vi "ESP30xCore.vi"(5 "NumOfAxis":i32=3, 6 "MotorDisabled":refnum<vi>, 7 "Simulation":bool, 8 "error in":errorcluster, 9 "Serial Configuration":T1={"Baud Rate"=19200, "Parity"=0, "Data Bits"=8, "Stop Bits"=10, "Flow Control"=2} {"Flow Control" items=["None", "XON/XOFF", "RTS/CTS", "XON/XOFF & RTS/CTS", "DTR/DSR", "XON/XOFF & DTR/DSR"]; "Stop Bits" items=["1.0"=10, "1.5"=15, "2.0"=20]; "Data Bits" items=["7"=7, "8"=8]; "Parity" items=["None", "Odd", "Even", "Mark", "Space"]; "Baud Rate" items=["300"=300, "600"=600, "1200"=1200, "2400"=2400, "4800"=4800, "9600"=9600, "19200"=19200]}, 10 "CommPort":refnum<visa-resource-name>="COM3", 11 "ControlQueue in":refnum<queue>) -> (0 "error out":errorcluster, 3 "queue out":refnum<queue>)   [LabVIEW 2013, in "ESP300.lvlib"]
uses:
  <instrlib>/ESP300/ESP300.lvlib
  <instrlib>/ESP300/Public/Data/ESP300_State.ctl
  <instrlib>/ESP300/Public/Data/ESP30x_Data.ctl
  <vilib>/Utility/error.llb/DialogType.ctl
  <instrlib>/Micos_uic/Public/Data/Micos_State.ctl
  <instrlib>/Micos_uic/Public/Data/Micos_Data.ctl
  <instrlib>/ESP300/Public/Position_ESP300.vi
  <instrlib>/Micos_uic/Micos_uic.lvlib
panel:
  in  "+Z_fine":bool
  in  "-Z_fine":bool
  in  "++Z":bool
  in  "--Z":bool
  in  "+Z":bool
  in  "-Z":bool
  out "WaitStopBlink":i32
  in  "StepWidth":dbl(ring)=0.2 items=["0.2 um"=0.0002, "0.001 mm"=0.001, "0.002 mm"=0.002, "0.005 mm "=0.005, "0.01 mm"=0.01, "0.02 mm"=0.02, "0.05 mm"=0.05, "0.1 mm"=0.1, "0.2 mm"=0.2, "1 mm"=1.0]
  in  "MotorDisabled":bool caption="Go"
  in  "Home":bool caption="Go"
  in  "Z-":bool
  in  "Z+":bool
  in  "X+":bool
  in  "X-":bool
  in  "Y-":bool
  in  "Y+":bool
  in  "ClearErr":bool caption="Go"
  in  "STOP":bool caption="Go"
  in  "Quit":bool caption="Go"
  out "Instrument Driver Revision":string
  out "Instrument Firmware Revision":string
  in  "SetPosition":dbl[](array[numeric])=[10.93352, 0.3355, 20.38401000000006] caption="Position" format="%.4f"
  in  "SetVelocity":dbl[](array[numeric])=[0.2, 0.2, 0.2] caption="Velocity"
  in  "SetAcceleration":dbl[](array[numeric])=[0.8, 0.8, 0.8] caption="Acceleration"
  in  "Go":bool
  out "Moving":bool
  out "Acceleration":dbl[](array[numeric])
  out "Velocity":dbl[](array[numeric])
  out "Position":dbl[](array[numeric])
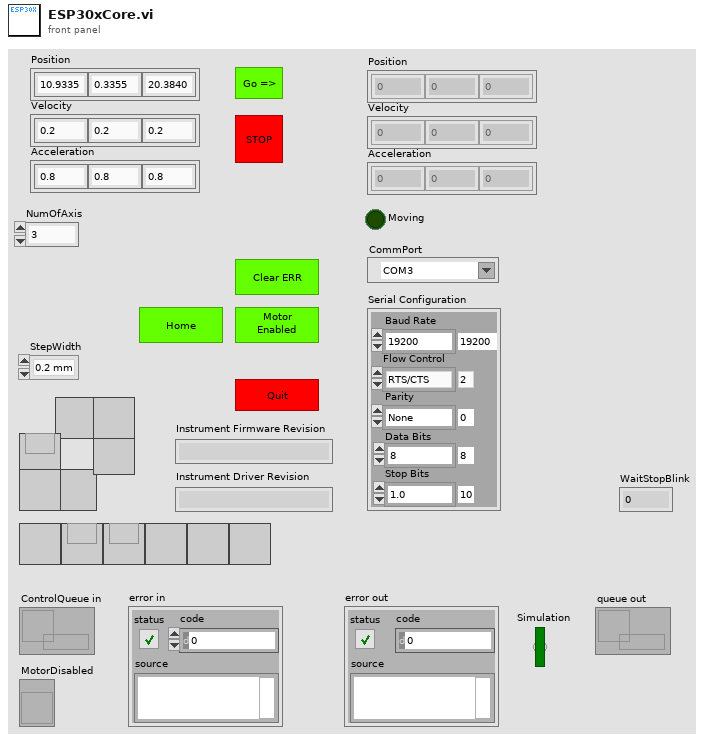
[diagram p1: front panel]
types:
  T1 = cluster{"Baud Rate":u32, "Parity":u16, "Data Bits":u16, "Stop Bits":u16, "Flow Control":u16}
  T2 = cluster{"CommPort":refnum<vi>, "Serial Configuration":refnum<vi>, "SetPosition":refnum<vi>, "SetAcceleration":refnum<vi>, "SetVelocity":refnum<vi>, "StepWidth":refnum<vi>}
  T3 = typedef "ESP300.lvlib/ESP300_State.ctl" = cluster{"State":enum16{"Initialize", "SetDefaultConfig", "Close", "Quit", "Identify", "MoveAbs", "MoveAbs_all", "MoveRel", "MoveRel_all", "STOP", "Origin/Home", "WaitStop", "QueryStatus", "UpdateXPos", "UpdateAll", "SetVelocity", "SetAcceleration", "ClearErr", "LogMessage", "MotorEnable(1)", "EnableAxis", "JoyStick", "GetVelocity", "GetAcceleration", "SendCmd", "SetSoftLimits", "Beep", "_SettingReturn", "SoftReset"}, "Params.":variant}
  T4 = typedef "ESP300.lvlib/ESP30x_Data.ctl" = cluster{"Position":dbl[], "Velocity":dbl[], "Acceleration":dbl[], "Moving":bool, "Simulation":bool, "tickcount_mov":u32, "tickcount_pos":u32, "NumOfAxis":i32, "Initialized":bool, "CommPort":refnum<visa-resource-name>, "Range":dbl[][], "Serial Configuration":cluster{"Baud Rate":u32, "Parity":u16, "Data Bits":u16, "Stop Bits":u16, "Flow Control":u16}, "MotorDisabled":refnum<vi>}
  T5 = cluster{"Acceleration":dbl[], "Velocity":dbl[], "JogSpeed":dbl[]}
  T6 = cluster{"Acceleration":dbl[], "Velocity":dbl[], "tick_move_target":u32, "Position target":dbl[], "Velocity_axial":dbl[]}
  T7 = cluster{"Position_Target":dbl[], "Velocity_axial":dbl[], "Acceleration":dbl[], "Moving":bool, "Simulation":bool, "tick_MoveTarget":u32, "NumOfAxis":i32, "Range":dbl[][]}
  T8 = typedef "Micos_uic.lvlib/Micos_State.ctl" = cluster{"State":enum16{"Initialize", "SetDefaultConfig", "Close", "Quit", "Identify", "MoveAbs", "MoveAbs_all", "MoveRel", "MoveRel_all", "STOP", "Origin/Home", "WaitStop", "QueryStatus", "UpdateXPos", "UpdateAll", "SetVelocity", "SetAcceleration", "ClearErr", "LogMessage", "MotorEnable(1)", "EnableAxis", "JoyStick", "GetVelocity", "GetAcceleration", "SendCmd", "SetSoftLimits", "Beep", "_SettingReturn", "SoftReset"}, "Params.":variant}
  T9 = typedef "Micos_uic.lvlib/Micos_Data.ctl" = cluster{"Position":dbl[], "Velocity":dbl[], "Acceleration":dbl[], "Moving":bool, "Simulation":bool, "tickcount_mov":u32, "tickcount_pos":u32, "NumOfAxis":i32, "Initialized":bool, "CommPort":refnum<visa-resource-name>, "Range":dbl[][], "Serial Configuration":cluster{"Baud Rate":u32, "Parity":u16, "Data Bits":u16, "Stop Bits":u16, "Flow Control":u16}, "MotorDisabled":refnum<vi>}
  T10 = enum16{"Initialize", "SetDefaultConfig", "Close", "Quit", "Identify", "MoveAbs", "MoveAbs_all", "MoveRel", "MoveRel_all", "STOP", "Origin/Home", "WaitStop", "QueryStatus", "UpdateXPos", "UpdateAll", "SetVelocity", "SetAcceleration", "ClearErr", "LogMessage", "MotorEnable(1)", "EnableAxis", "JoyStick", "GetVelocity", "GetAcceleration", "SendCmd", "SetSoftLimits", "Beep", "_SettingReturn"}
  T11 = typedef "DialogType.ctl" = u16
  T12 = enum16{"Initialize", "SetDefaultConfig", "Close", "Quit", "Identify", "MoveAbs", "MoveAbs_all", "MoveRel", "MoveRel_all", "STOP", "Origin/Home", "WaitStop", "QueryStatus", "UpdateXPos", "UpdateAll", "SetVelocity", "SetAcceleration", "ClearErr", "LogMessage", "MotorEnable(1)", "EnableAxis", "JoyStick", "GetVelocity", "GetAcceleration", "SendCmd", "SetSoftLimits", "Beep", "_SettingReturn", "SoftReset"}
  T13 = enum16{"Initialize", "SetDefaultConfig", "Close", "Quit", "Identify", "MoveAbs", "MoveAbs_all", "MoveRel", "MoveRel_all", "STOP", "Origin/Home", "WaitStop", "QueryStatus", "UpdateXPos", "UpdateAll", "SetVelocity", "SetAcceleration", "ClearErr", "LogMessage", "MotorEnable(1)", "EnableAxis", "JoyStick", "GetVelocity", "GetAcceleration", "SendCmd", "SetSoftLimits", "Beep", "_SettingReturn"}[]
  T14 = typedef "StepWidthSelector.ctl" = dbl
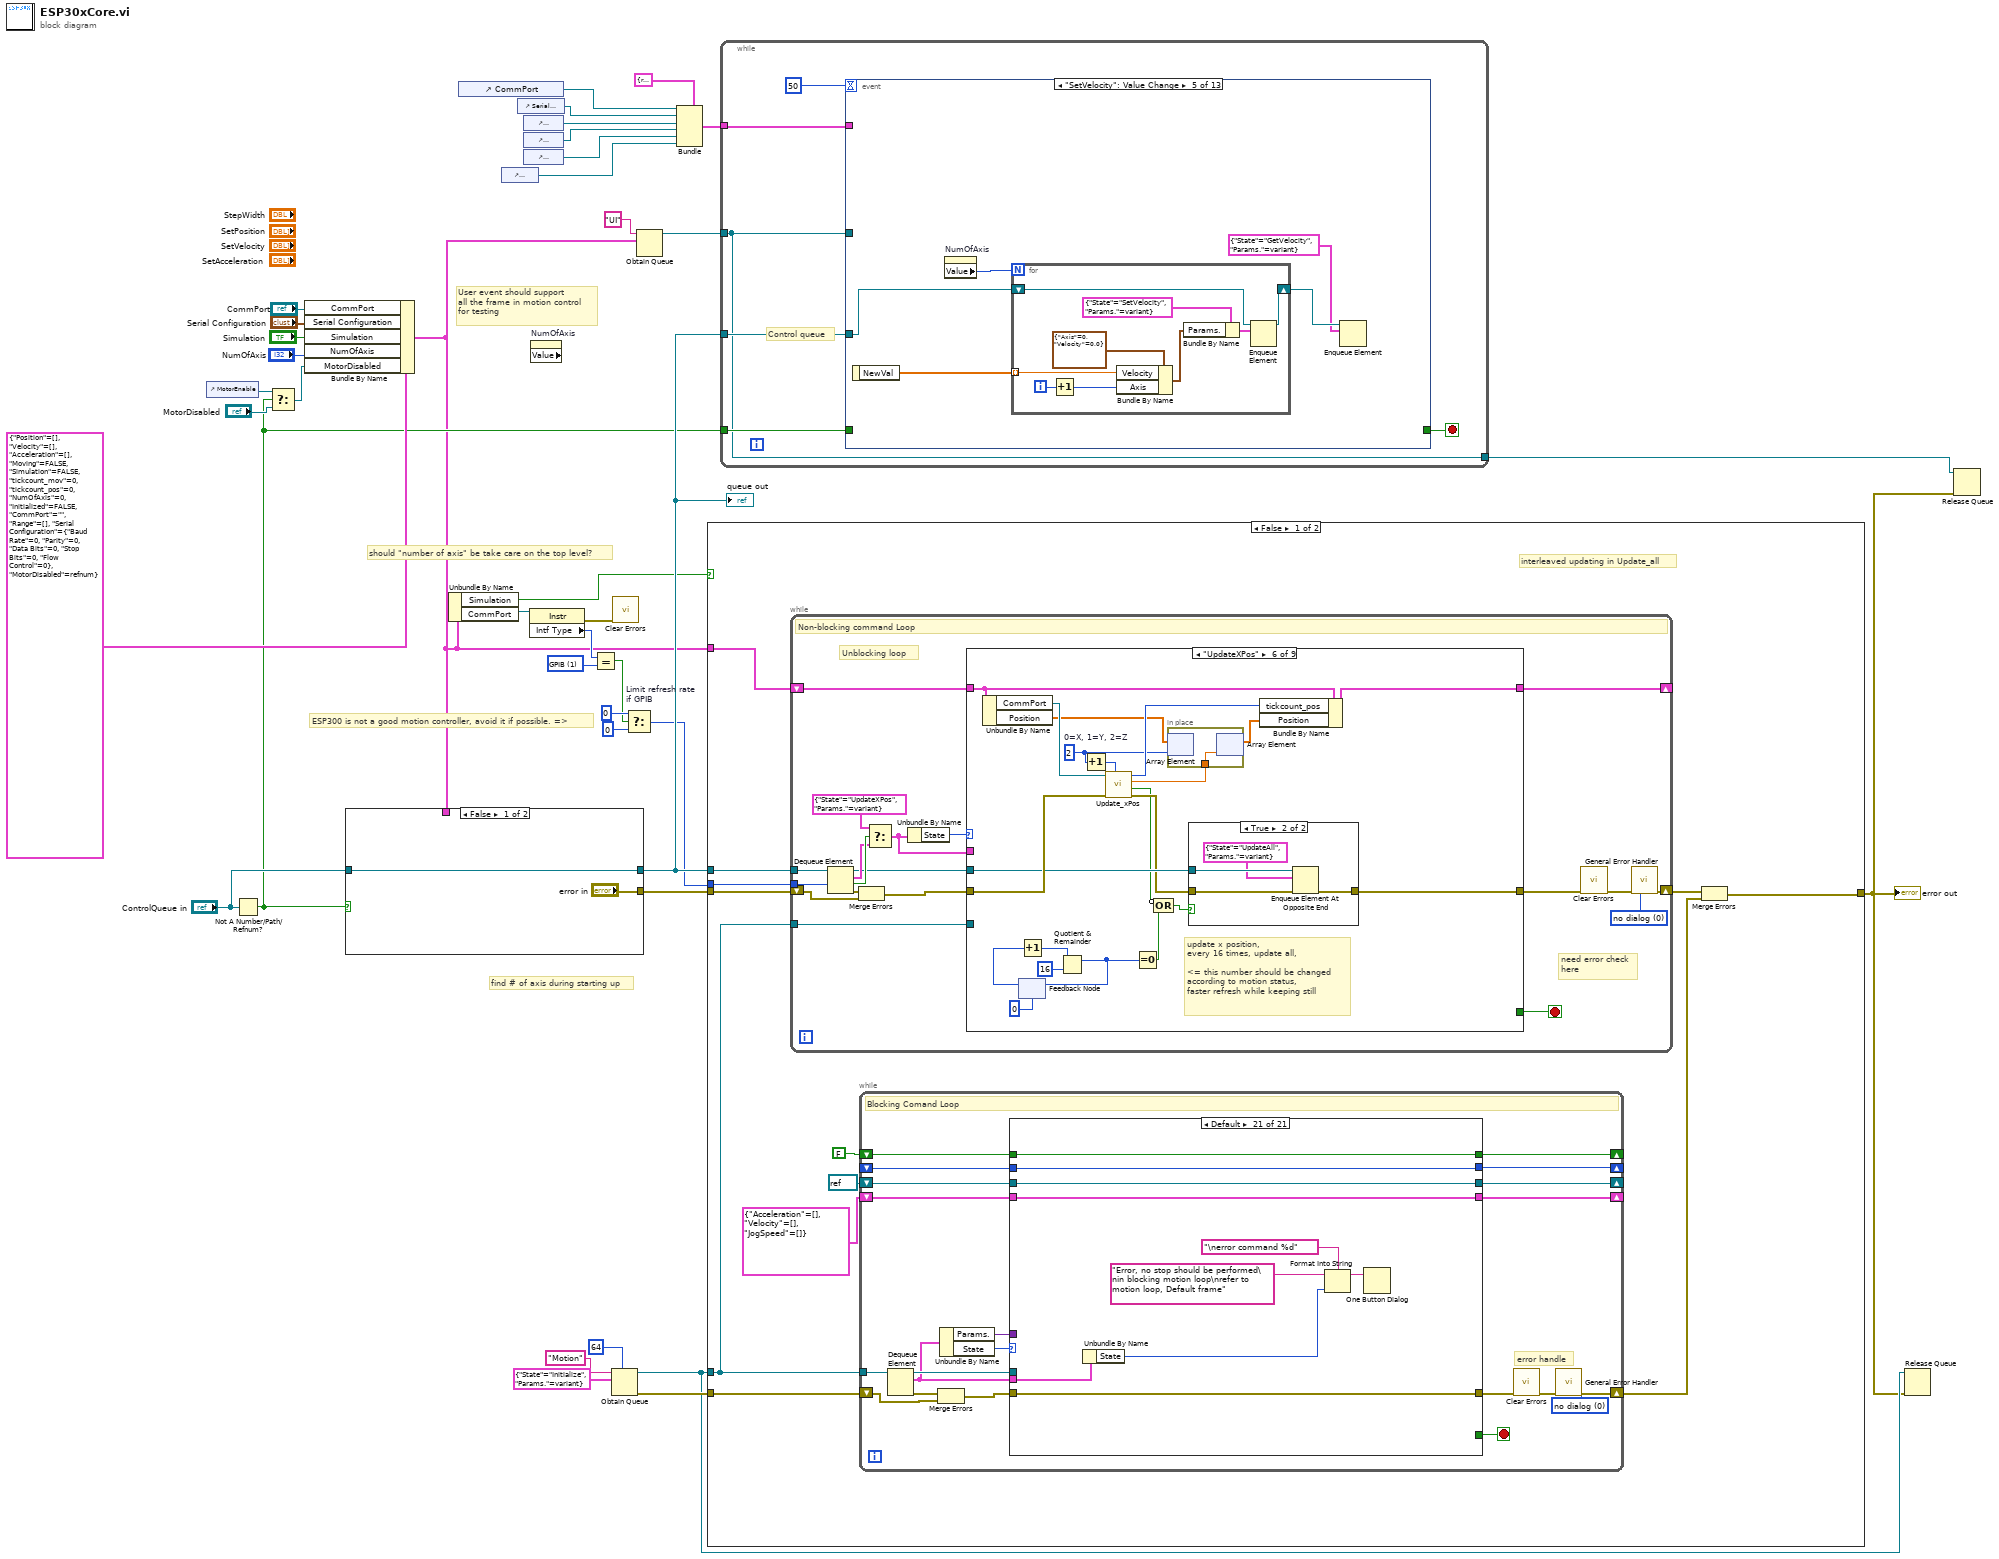
[diagram p0: block diagram]
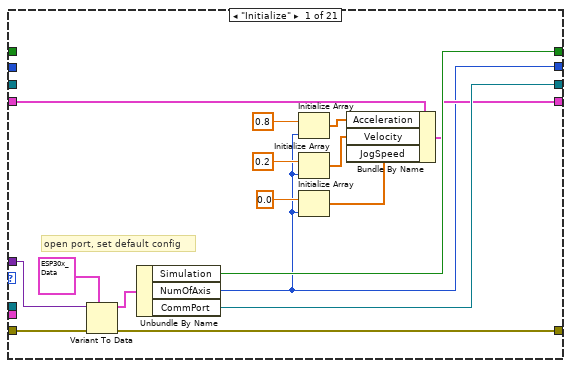
[diagram p2: hidden frame]
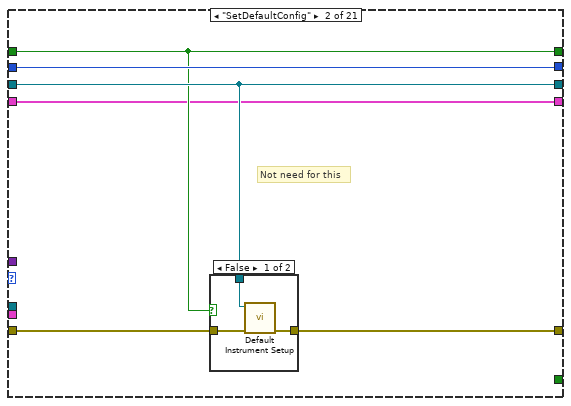
[diagram p3: hidden frame]
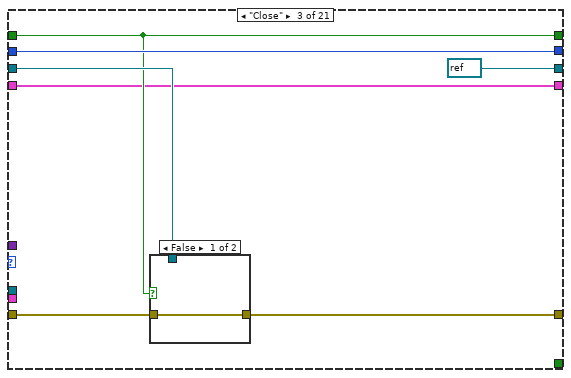
[diagram p5: hidden frame]
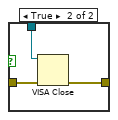
[diagram p6: hidden frame]
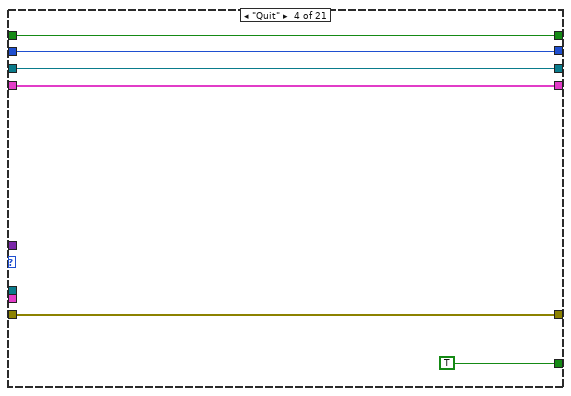
[diagram p7: hidden frame]
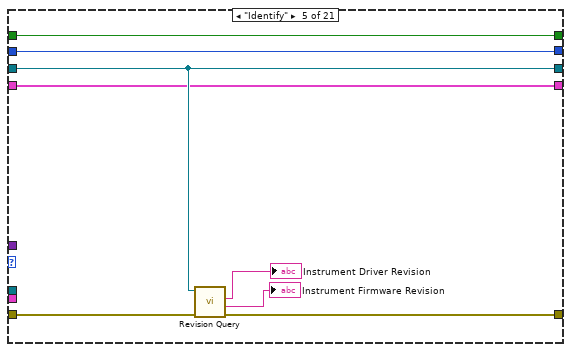
[diagram p8: hidden frame]
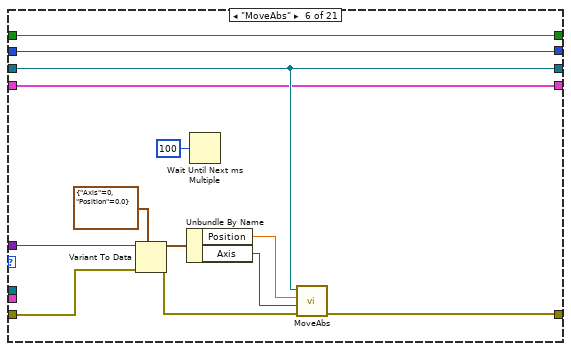
[diagram p9: hidden frame]
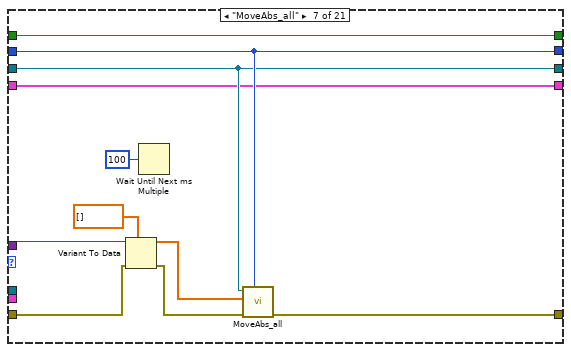
[diagram p10: hidden frame]
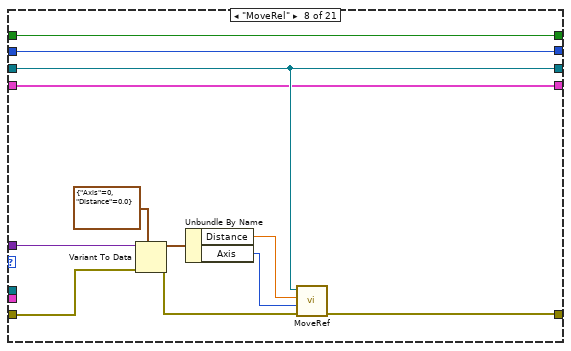
[diagram p11: hidden frame]
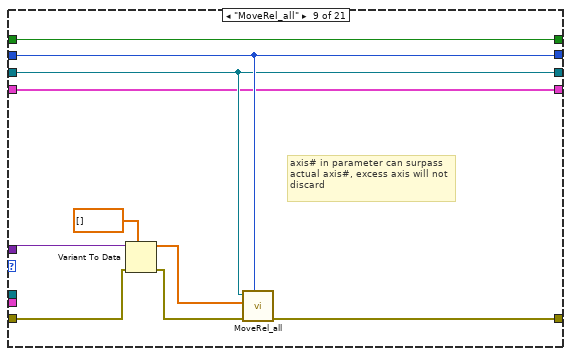
[diagram p12: hidden frame]
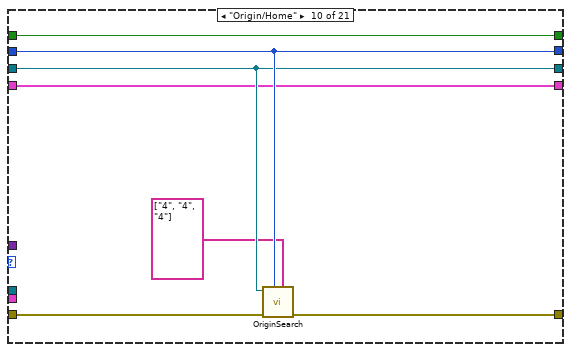
[diagram p13: hidden frame]
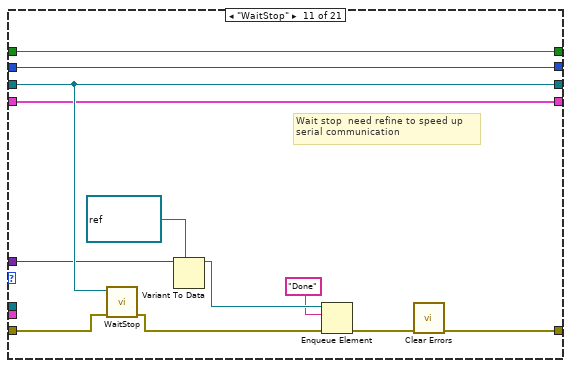
[diagram p14: hidden frame]
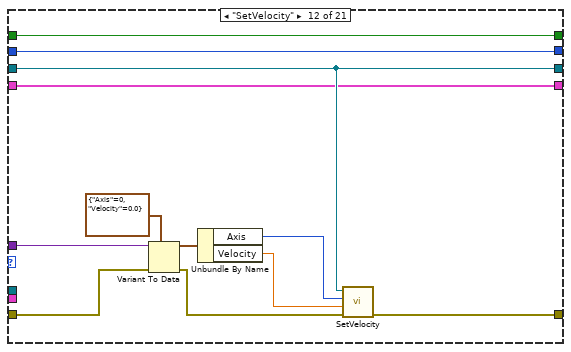
[diagram p15: hidden frame]
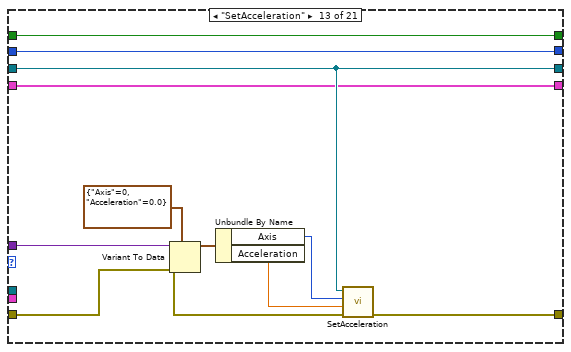
[diagram p16: hidden frame]
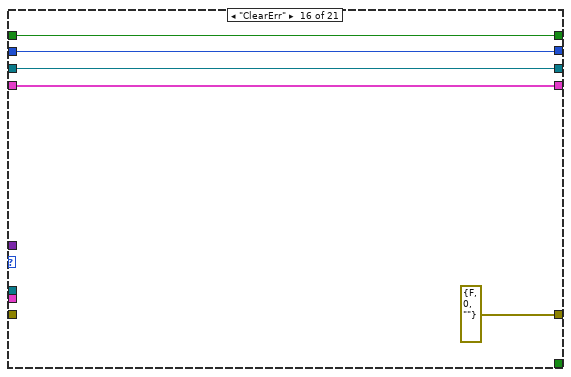
[diagram p19: hidden frame]
diagram:
  w14 = u16 1 items=["GPIB"=1, "VXI"=2, "GPIB-VXI"=3, "Serial"=4, "PXI"=5, "TCPIP"=6, "USB"=7, "FireWire"=9] ("Interface Information:Interface Type")
  # "ESP300 is not a good motion controller, avoid it if possible. =>"
  # "find # of axis during starting up"
  # "User event should support \nall the frame in motion control\nfor testing"
  # "should \"number of axis\" be take care on the top level?"
  n1 = control-ref of="MotorEnable"() -> (w12:refnum<vi>)
  n2 = Not A Number/Path/Refnum?(number/path/refnum="ControlQueue in") -> (NaN/Path/Refnum?=w10:bool)
  n3 = Select(t=w12, s=w10, f="MotorDisabled") -> (s? t:f=w9:refnum<vi>)
  n4 = Bundle By Name(cluster=T4 {"Position"=[], "Velocity"=[], "Acceleration"=[], "Moving"=FALSE, "Simulation"=FALSE, "tickcount_mov"=0, "tickcount_pos"=0, "NumOfAxis"=0, "Initialized"=FALSE, "CommPort"="", "Range"=[], "Serial Configuration"={"Baud Rate"=0, "Parity"=0, "Data Bits"=0, "Stop Bits"=0, "Flow Control"=0}, "MotorDisabled"=refnum}, "CommPort"="CommPort", "Serial Configuration"="Serial Configuration", "Simulation"="Simulation", "NumOfAxis"="NumOfAxis", "MotorDisabled"=w9) -> (w8:T4)
  n5 = case shown="False" w10 {
    tunnel: [w41 w47] -> w37
    tunnel: ["error in" w46] -> w39
    tunnel: "ControlQueue in" -> [w41 _]
    tunnel: w8 -> [_ w43]
    frame False {
    }
    frame True {
      w48 = T3 {"State"=enum."Initialize", "Params."=variant}
      # "Control queue invalid, \nassume standalone program"
      n6 = Bundle By Name(cluster=w48, "Params."=w43) -> (w44:T3)
      n7 = Obtain Queue(name (unnamed)="Control", element data type=w48) -> (queue out=w49:refnum<queue>, error out=w45:errorcluster)  [unwired: 3 in, 1 out]
      n8 = Enqueue Element(queue=w49, element=w44, error in (no error)=w45) -> (queue out=w47:refnum<queue>, error out=w46:errorcluster)  [unwired: 1 in, 1 out]
    }
  }
  "queue out" <- w37
  n9 = Unbundle By Name(w8) -> ("Simulation"=w5:bool, "CommPort"=w16:refnum<visa-resource-name>)
  n10 = control-ref of="CommPort"() -> (w29:refnum<vi>)
  n11 = control-ref of="StepWidth"() -> (w6:refnum<vi>)
  n12 = control-ref of="Serial Configuration"() -> (w30:refnum<vi>)
  n13 = control-ref of="SetPosition"() -> (w28:refnum<vi>)
  n14 = control-ref of="SetAcceleration"() -> (w27:refnum<vi>)
  n15 = control-ref of="SetVelocity"() -> (w26:refnum<vi>)
  n16 = property class="Instr"(reference=w16) -> (error out=w7:errorcluster, "Intf Type"=w15:u16)  [unwired: 1 in, 1 out]
  n17 = property on="NumOfAxis" class="DigNum (strict)" props=["Value"]() -> ()  [unwired: 2 in, 3 out]
  n18 = Equal?(x=w15, y=w14) -> (x = y?=w13:bool)
  n19 = Obtain Queue(max queue size (-1, unlimited)=64, name (unnamed)="Motion", element data type=T3 {"State"=enum."Initialize", "Params."=variant}) -> (queue out=w4:refnum<queue>, error out=w35:errorcluster)  [unwired: 2 in, 1 out]
  n20 = call <vilib>:"Clear Errors.vi"("error in (no error)"=w7) -> ()  [unwired: 6 in, 1 out]
  n21 = Select "Limit refresh rate \nif GPIB"(t=0 ("timeout in ms (-1)"), s=w13, f=0) -> (s? t:f=w17:i32)
  n22 = Obtain Queue(name (unnamed)="UI", element data type=w8) -> (queue out=w3:refnum<queue>)  [unwired: 3 in, 2 out]
  n23 = Bundle(cluster=T2 {"CommPort"=refnum, "Serial Configuration"=refnum, "SetPosition"=refnum, "SetAcceleration"=refnum, "SetVelocity"=refnum, "StepWidth"=refnum}, "CommPort"=w29, "Serial Configuration"=w30, "SetPosition"=w28, "SetAcceleration"=w27, "SetVelocity"=w26, "StepWidth"=w6) -> (w25:T2)
  n24 = case shown="False" w5 {
    tunnel: w39 -> [w61 w490]
    tunnel: w37 -> [w60 w496]
    tunnel: w35 -> [w59 w494]
    tunnel: w4 -> [w58 w495]
    tunnel: w17 -> [w54 _]
    tunnel: w8 -> [w53 w497]
    tunnel: [w51 w488] -> w2
    frame False {
      # "interleaved updating in Update_all"
      n25 = while {
        tunnel: w60 -> [w310]
        shift-right: [w322] -> _
        shift-left: w53 -> [w321]
        tunnel: w58 -> [w319]
        shift-right: [w313] -> w55
        shift-left: w61 -> [w305]
        tunnel: w54 -> [w307]
        stop <- w320 stop-if-true
        w312 = T11 0 items=["no dialog", "OK message", "continue or stop message", "OK message + warnings", "continue/stop + warnings"] ("type of dialog (OK msg:1)")
        # "Unblocking loop"
        # "need error check\nhere"
        # "Non-blocking command Loop"
        n26 = Dequeue Element(queue=w310, timeout in ms (-1)=w307) -> (queue out=w311:refnum<queue>, element=w315:T3, timed out?=w317:bool, error out=w318:errorcluster)  [unwired: 1 in]
        n27 = Merge Errors(w318, w305) -> (w306:errorcluster)
        n28 = Select(t=T3 {"State"=enum."UpdateXPos", "Params."=variant} ("element"), s=w317, f=w315) -> (s? t:f=w314:T3)
        n29 = Unbundle By Name(w314) -> ("State"=w309:T12)
        n30 = case shown="\"UpdateXPos\"" w309 {
          tunnel: w314 -> [w330 w357 _ _ w426 _ _ _ w473]
          tunnel: [w339 w362 w381 w396 w423 w449 w467 w469 w478] -> w322
          tunnel: w321 -> [w333 w360 w381 w396 w423 w447 w465 w469 w478]
          tunnel: [w329 _ TRUE _ _ _ _ _ _] -> w320
          tunnel: w319 -> [w323 w365 w384 w408 _ _ _ _ w477]
          tunnel: [w332 w363 w386 w405 w421 w436 w456 errorcluster {"status"=FALSE, "code"=0, "source"=""} ("error out") w470] -> w308
          tunnel: w306 -> [w336 w364 w382 w407 w422 w448 w466 _ w476]
          tunnel: w311 -> [_ w358 _ _ _ w435 _ _ w474]
          frame "Initialize" {
            # "cmd +(stage data)"
            # "stage data"
            n31 = Unbundle By Name(w330) -> ("Params."=w337:variant)
            n32 = Variant To Data(error in=w336, type=w333, Variant=w337) -> (data=w334:T4, error out=w335:errorcluster)
            n33 = Select(t=w333, s=w335, f=w334) -> (s? t:f=w325:T4)
            n34 = Unbundle By Name(w325) -> ("Serial Configuration"=w331:T1, "CommPort"=w327:refnum<visa-resource-name>)
            n35 = call <vilib>:"Clear Errors.vi"("error in (no error)"=w335) -> ("error out"=w324:errorcluster)  [unwired: 6 in]
            n36 = Equal?(x=w327, y=refnum<visa-resource-name> refnum ("CommPort")) -> (x = y?=w328:bool)
            n37 = Bundle By Name(cluster=w325, "Initialized"=TRUE) -> (w339:T4)
            n38 = case shown="False" w328 {
              tunnel: w324 -> [w350 w353]
              tunnel: [w341 errorcluster {"status"=FALSE, "code"=-5104, "source"="Device unspecifiied,\nSkip execution"} ("error out")] -> w332
              tunnel: w331 -> [w349 _]
              tunnel: w327 -> [w348 _]
              tunnel: [_ TRUE] -> w329
              tunnel: w325 -> [w343 _]
              tunnel: w323 -> [w340 w351]
              frame False {
                n39 = Bundle By Name(cluster=T3 {"State"=enum."Initialize", "Params."=variant}, "Params."=w343) -> (w345:T3)
                n40 = call <instrlib>:"Initialize.vi"("Serial Configuration"=w349, "error in (no error)"=w350, "Reset (True)"=FALSE, "ID Query (True)"=FALSE, "VISA resource name"=w348) -> ("error out"=w342:errorcluster)  [unwired: 5 in, 1 out]
                n41 = Enqueue Element(queue=w340, element=w345, error in (no error)=w342) -> (error out=w341:errorcluster)  [unwired: 1 in, 2 out]
              }
              frame True {
                n42 = property on="Quit" class="Bool (strict)"("Val(Sgnl)"=TRUE ("Value (Signaling)")) -> ()  [unwired: 2 in, 2 out]
                n43 = Enqueue Element(queue=w351, element=T3 {"State"=enum."Quit", "Params."=variant}, error in (no error)=w353) -> ()  [unwired: 1 in, 3 out]
              }
            }
          }
          frame "Close" {
            n44 = Unbundle By Name(w360) -> ("Moving"=w359:bool)
            n45 = case shown="True" w359 {
              tunnel: w365 -> [w369 _]
              tunnel: w364 -> [w368 w374]
              tunnel: [w367 w371] -> w363
              tunnel: w358 -> [_ w379]
              tunnel: w357 -> [w366 w370]
              frame False {
                n46 = Enqueue Element "Imply Close"(queue=w369, element=w366, error in (no error)=w368) -> (error out=w367:errorcluster)  [unwired: 1 in, 2 out]
              }
              frame True {
                n47 = Enqueue Element At Opposite End "Imply Close"(queue=w379, element=w370, error in (no error)=w374) -> (queue out=w378:refnum<queue>, error out=w373:errorcluster)  [unwired: 1 in, 1 out]
                n48 = Enqueue Element At Opposite End(queue=w378, element=T3 {"State"=enum."UpdateAll", "Params."=variant}, error in (no error)=w373) -> (queue out=w377:refnum<queue>, error out=w372:errorcluster)  [unwired: 1 in, 1 out]
                n49 = Enqueue Element At Opposite End(queue=w377, element=T3 {"State"=enum."STOP", "Params."=variant}, error in (no error)=w372) -> (error out=w371:errorcluster)  [unwired: 1 in, 2 out]
              }
            }
            n50 = Bundle By Name(cluster=w360, "Initialized"=FALSE) -> (w362:T4)
          }
          frame "Quit" {
            n51 = Unbundle By Name(w381) -> ("Initialized"=w380:bool)
            n52 = case shown="True" w380 {
              tunnel: [w390 w394] -> w385
              tunnel: w384 -> [w390 w393]
              tunnel: [w389 w392] -> w383
              tunnel: w382 -> [w389 w391]
              frame False {
              }
              frame True {
                n53 = Enqueue Element(queue=w393, element=T3 {"State"=enum."Close", "Params."=variant}, error in (no error)=w391) -> (queue out=w394:refnum<queue>, error out=w392:errorcluster)  [unwired: 1 in, 1 out]
              }
            }
            n54 = Enqueue Element(queue=w385, element=T3 {"State"=enum."Quit", "Params."=variant}, error in (no error)=w383) -> (error out=w386:errorcluster)  [unwired: 1 in, 2 out]
          }
          frame "STOP" {
            w401 = T13 [enum."WaitStop", enum."UpdateAll", enum."Close", enum."Quit", enum."SetVelocity"] items=["Initialize", "SetDefaultConfig", "Close", "Quit", "Identify", "MoveAbs", "MoveAbs_all", "MoveRel", "MoveRel_all", "STOP", "Origin/Home", "WaitStop", "QueryStatus", "UpdateXPos", "UpdateAll", "SetVelocity", "SetAcceleration", "ClearErr", "LogMessage", "MotorEnable(1)", "EnableAxis", "JoyStick", "GetVelocity", "GetAcceleration", "SendCmd", "SetSoftLimits", "Beep", "_SettingReturn"]
            # "send stop to controller, update"
            n55 = Flush Queue(queue=w408, error in (no error)=w407) -> (queue out=w400:refnum<queue>, remaining elements=w399:T3[], error out=w406:errorcluster)
            n56 = Unbundle By Name(w396) -> ("CommPort"=w403:refnum<visa-resource-name>)
            n57 = for {
              tunnel: w399 -> [w416] mode=indexing
              tunnel: w401 -> [w413]
              shift-right: [w414] -> w398
              shift-left: w400 -> [w415]
              n58 = Unbundle By Name(w416) -> ("State"=w412:T12)
              n59 = Search 1D Array(1D array=w413, element=w412) -> (index of element=w411:i32)  [unwired: 1 in]
              n60 = Not Equal?(x=w411, y=-1) -> (x != y?=w410:bool)
              n61 = case shown="True" w410 {
                tunnel: w416 -> [_ w420]
                tunnel: w415 -> [w417 w419]
                tunnel: [w417 w418] -> w414
                frame False {
                }
                frame True {
                  n62 = Enqueue Element At Opposite End(queue=w419, element=w420) -> (queue out=w418:refnum<queue>)  [unwired: 2 in, 2 out]
                }
              }
            }
            n63 = call <instrlib>:"VISA_Write+Read.vi"("Read?(T)"=FALSE, "error in (no error)"=w406, "Write Buffer"="ST" ("write buffer"), "VISA resource name"=w403) -> ("error out"=w405:errorcluster)  [unwired: 5 in, 2 out]
            n64 = Enqueue Element At Opposite End(queue=w398, element=T3 {"State"=enum."STOP", "Params."=variant}) -> ()  [unwired: 2 in, 3 out]
          }
          frame "QueryStatus" {
            # "return the value to queue"
            n65 = Unbundle By Name(w426) -> ("Params."=w428:variant)
            n66 = Variant To Data(error in=w422, type=refnum<queue> refnum ("queue out"), Variant=w428) -> (data=w425:refnum<queue>, error out=w427:errorcluster)
            n67 = Enqueue Element(queue=w425, element=w423, error in (no error)=w427) -> (error out=w421:errorcluster)  [unwired: 1 in, 2 out]
          }
          frame "UpdateXPos" {
            w429 = 2  # 0=X, 1=Y, 2=Z
            # "update x position,\nevery 16 times, update all,\n\n<= this number should be changed \naccording to motion status, \nfaster refresh while keeping still"
            n68 = Unbundle By Name(w447) -> ("CommPort"=w446:refnum<visa-resource-name>, "Position"=w444:dbl[])
            n69 = feedback #1(0) -> (w439:i32)
            n70 = Increment(x=w439) -> (x+1=w440:i32)
            n71 = Quotient & Remainder(x=w440, y=16) -> (x-y*floor(x/y)=w437:i32)  [unwired: 1 out]
            n72 = feedback-in #1(w437) -> ()
            n73 = Increment(x=w429) -> (x+1=w430:i32)
            n74 = call <instrlib>:"Update_xPos.vi"("FastUpdateAxis"=w430, "error in (no error)"=w448, "VISA resource name"=w446) -> ("error out"=w434:errorcluster, "x_Moving"=w431:bool, "x_pos"=w442:dbl, "tickcount_pos"=w445:u32)  [unwired: 5 in]
            n75 = Equal To 0?(x=w437) -> (x = 0?=w433:bool)
            n76 = Compound Arithmetic op=OR(invert w431, w433) -> (w432:bool)
            n77 = in-place {
              in-place-border: w442 -> [w455]
              n78 = in-place-array #2(w444, w429) -> ()  [unwired: 1 out]
              n79 = in-place-array #2(w455) -> (w443:dbl[])  [unwired: 1 out]
            }
            n80 = case shown="True" w432 {
              tunnel: [w450 w454] -> w436
              tunnel: w435 -> [_ w453]
              tunnel: w434 -> [w450 w451]
              frame False {
              }
              frame True {
                n81 = Enqueue Element At Opposite End(queue=w453, element=T3 {"State"=enum."UpdateAll", "Params."=variant}, error in (no error)=w451) -> (error out=w454:errorcluster)  [unwired: 1 in, 2 out]
              }
            }
            n82 = Bundle By Name(cluster=w447, "tickcount_pos"=w445, "Position"=w443) -> (w449:T4)
          }
          frame "UpdateAll" {
            n83 = Unbundle By Name(w465) -> ("NumOfAxis"=w464:i32, "CommPort"=w463:refnum<visa-resource-name>, "MotorDisabled"=w459:refnum<vi>)
            n84 = call <instrlib>:"Update_all.vi"("# axis"=w464, "error in (no error)"=w466, "VISA resource name"=w463) -> ("error out"=w457:errorcluster, "Moving"=w460:bool, "Currrent postion"=w461:dbl[], "tickcount_pos"=w462:u32, "MotorDisabled"=w458:bool)  [unwired: 4 in]
            n85 = property class="Bool (strict)"(reference=w459, error in=w457, "Value"=w458, "Blinking"=w458) -> (error out=w456:errorcluster)  [unwired: 1 out]
            n86 = Bundle By Name(cluster=w465, "tickcount_pos"=w462, "Position"=w461, "Moving"=w460) -> (w467:T4)
          }
          frame "ClearErr" {
          }
          frame Default {
            # "timeout push command back then do update?\n\npreventing blocking"
            n87 = Enqueue Element(queue=w477, element=w473, timeout in ms (-1)=0, error in (no error)=w476) -> (timed out?=w471:bool, error out=w472:errorcluster)  [unwired: 1 out]
            n88 = case shown="True" w471 {
              tunnel: w474 -> [_ w486]
              tunnel: w473 -> [_ w485]
              tunnel: w472 -> [w479 w484]
              tunnel: [w479 w481] -> w470
              frame False {
              }
              frame True {
                n89 = Enqueue Element At Opposite End(queue=w486, element=w485, error in (no error)=w484) -> (queue out=w483:refnum<queue>, error out=w480:errorcluster)  [unwired: 1 in, 1 out]
                n90 = Enqueue Element At Opposite End(queue=w483, element=T3 {"State"=enum."UpdateXPos", "Params."=variant}, error in (no error)=w480) -> (error out=w481:errorcluster)  [unwired: 1 in, 2 out]
              }
            }
          }
        }
        n91 = call <vilib>:"Clear Errors.vi"("error in (no error)"=w308) -> ("error out"=w304:errorcluster)  [unwired: 6 in]
        n92 = call <vilib>:"General Error Handler.vi"("type of dialog (OK msg:1)"=w312, "error in (no error)"=w304) -> ("error out"=w313:errorcluster)  [unwired: 9 in, 4 out]
      }
      n93 = while {
        tunnel: w58 -> [w82]
        shift-right: [w74] -> w52
        shift-left: w59 -> [w63]
        shift-right: [w78] -> _
        shift-left: refnum<visa-resource-name> refnum ("CommPort") -> [w77]
        shift-right: [w72] -> _
        shift-left: _ -> [w71]
        shift-right: [w68] -> _
        shift-left: FALSE -> [w69]
        shift-right: [w66] -> _
        shift-left: T5 {"Acceleration"=[], "Velocity"=[], "JogSpeed"=[]} -> [w65]
        stop <- w81 stop-if-true
        w73 = T11 0 items=["no dialog", "OK message", "continue or stop message", "OK message + warnings", "continue/stop + warnings"] ("type of dialog (OK msg:1)")
        # "error handle"
        # "Blocking Comand Loop"
        n94 = Dequeue Element(queue=w82) -> (queue out=w76:refnum<queue>, element=w75:T3, error out=w79:errorcluster)  [unwired: 2 in, 1 out]
        n95 = Merge Errors(w79, w63) -> (w64:errorcluster)
        n96 = Unbundle By Name(w75) -> ("Params."=w70:variant, "State"=w62:T12)
        n97 = case shown="Default" w62 {
          tunnel: w75 -> [_ _ _ _ _ _ _ _ _ _ _ _ _ _ _ _ _ _ _ _ w298]
          tunnel: [_ _ _ TRUE _ _ _ _ _ _ _ _ _ _ _ _ _ _ _ _ _] -> w81
          tunnel: [w97 w102 w113 w120 w130 w144 w157 w167 w179 w182 w189 w205 w217 w227 w232 errorcluster {"status"=FALSE, "code"=0, "source"=""} ("error out") w242 w251 w258 w274 w302] -> w80
          tunnel: w64 -> [w98 w103 w114 w120 w131 w141 w150 w164 w172 w183 w196 w207 w219 w227 w232 _ w242 w250 w259 w273 w302]
          tunnel: [w94 w101 refnum<visa-resource-name> refnum ("CommPort") w124 w129 w143 w155 w166 w177 w184 w194 w209 w221 w226 w231 w236 w241 w246 w255 w282 w303] -> w78
          tunnel: w77 -> [_ w101 w115 w124 w129 w143 w155 w166 w177 w184 w194 w209 w221 w226 w231 w236 w241 w246 w255 w282 w303]
          tunnel: w76 -> [_ _ _ _ _ _ _ _ _ _ _ _ _ _ _ _ _ _ _ w277 _]
          tunnel: [w83 w104 w111 w123 w133 w146 w156 w169 w178 w185 w198 w210 w222 w225 w230 w235 w240 w247 w264 w272 w301] -> w72
          tunnel: w71 -> [_ w104 w111 w123 w133 w146 w156 w169 w178 w185 w198 w210 w222 w225 w230 w235 w240 w247 w264 w272 w301]
          tunnel: w70 -> [w89 _ _ _ _ w142 w153 w165 w175 _ w193 w208 w220 _ _ _ _ w248 w262 _ _]
          tunnel: w69 -> [_ w100 w110 w122 w132 w145 w154 w168 w176 w186 w197 w204 w216 w224 w229 w234 w239 w252 w263 w281 w300]
          tunnel: [w93 w100 w110 w122 w132 w145 w154 w168 w176 w186 w197 w204 w216 w224 w229 w234 w239 w252 w263 w281 w300] -> w68
          tunnel: [w91 w99 w109 w121 w126 w134 w147 w158 w170 w181 w187 w199 w211 w223 w228 w233 w238 w243 w253 w280 w294] -> w66
          tunnel: w65 -> [w92 w99 w109 w121 w126 w134 w147 w158 w170 w181 w187 w199 w211 w223 w228 w233 w238 w243 w254 w276 w294]
          frame "Initialize" {
            # "open port, set default config"
            n98 = Variant To Data(error in=w98, type=T4 {"Position"=[], "Velocity"=[], "Acceleration"=[], "Moving"=FALSE, "Simulation"=FALSE, "tickcount_mov"=0, "tickcount_pos"=0, "NumOfAxis"=0, "Initialized"=FALSE, "CommPort"="", "Range"=[], "Serial Configuration"={"Baud Rate"=0, "Parity"=0, "Data Bits"=0, "Stop Bits"=0, "Flow Control"=0}, "MotorDisabled"=refnum}, Variant=w89) -> (data=w95:T4, error out=w97:errorcluster)
            n99 = Unbundle By Name(w95) -> ("Simulation"=w93:bool, "NumOfAxis"=w83:i32, "CommPort"=w94:refnum<visa-resource-name>)
            n100 = Initialize Array(0.8 ("element"), w83) -> (w88:dbl[])
            n101 = Initialize Array(0.2 ("element"), w83) -> (w87:dbl[])
            n102 = Initialize Array(0.0 ("element"), w83) -> (w86:dbl[])
            n103 = Bundle By Name(cluster=w92, "Acceleration"=w88, "Velocity"=w87, "JogSpeed"=w86) -> (w91:T5)
          }
          frame "SetDefaultConfig" {
            # "Not need for this"
            n104 = case shown="False" w100 {
              tunnel: w103 -> [w107 w108]
              tunnel: [w106 w108] -> w102
              tunnel: w101 -> [w105 _]
              frame False {
                n105 = call <instrlib>:"Default Instrument Setup.vi"("error in (no error)"=w107, "VISA resource name"=w105) -> ("error out"=w106:errorcluster)  [unwired: 8 in, 1 out]
              }
              frame True {
              }
            }
          }
          frame "Close" {
            n106 = case shown="False" w110 {
              tunnel: w115 -> [_ w119]
              tunnel: w114 -> [w116 w118]
              tunnel: [w116 w117] -> w113
              frame False {
              }
              frame True {
                n107 = VISA Close(VISA resource name=w119, error in (no error)=w118) -> (error out=w117:errorcluster)
              }
            }
          }
          frame "Quit" {
          }
          frame "Identify" {
            n108 = call <instrlib>:"Revision Query.vi"("error in (no error)"=w131, "VISA resource name"=w129) -> ("error out"=w130:errorcluster, "Instrument Firmware Revision"=→"Instrument Firmware Revision":string, "Instrument Driver Revision"=→"Instrument Driver Revision":string)  [unwired: 6 in, 1 out]
          }
          frame "MoveAbs" {
            n109 = Variant To Data(error in=w141, type=cluster{"Axis":i32, "Position":dbl} {"Axis"=0, "Position"=0.0}, Variant=w142) -> (data=w138:cluster{"Axis":i32, "Position":dbl}, error out=w140:errorcluster)
            n110 = Unbundle By Name(w138) -> ("Position"=w136:dbl, "Axis"=w137:i32)
            n111 = Wait Until Next ms Multiple(millisecond multiple=u32 100) -> ()  [unwired: 1 out]
            n112 = call <instrlib>:"MoveAbs.vi"("error in"=w140, "Axis"=w137, "Position"=w136, "VISA resource"=w143) -> ("error out"=w144:errorcluster)  [unwired: 7 in]
          }
          frame "MoveAbs_all" {
            n113 = Variant To Data(error in=w150, type=dbl[] [] ("Position"), Variant=w153) -> (data=w152:dbl[], error out=w149:errorcluster)
            n114 = Wait Until Next ms Multiple(millisecond multiple=u32 100) -> ()  [unwired: 1 out]
            n115 = call <instrlib>:"MoveAbs_all.vi"("# axis"=w156, "error in (no error)"=w149, "Position"=w152, "VISA resource name"=w155) -> ("error out"=w157:errorcluster)  [unwired: 7 in]
          }
          frame "MoveRel" {
            n116 = Variant To Data(error in=w164, type=cluster{"Axis":i32, "Distance":dbl} {"Axis"=0, "Distance"=0.0}, Variant=w165) -> (data=w161:cluster{"Axis":i32, "Distance":dbl}, error out=w163:errorcluster)
            n117 = Unbundle By Name(w161) -> ("Distance"=w159:dbl, "Axis"=w160:i32)
            n118 = call <instrlib>:"MoveRef.vi"("error in"=w163, "Axis"=w160, "Position"=w159, "VISA resource"=w166) -> ("error out"=w167:errorcluster)  [unwired: 7 in]
          }
          frame "MoveRel_all" {
            # "axis# in parameter can surpass\nactual axis#, excess axis will not\ndiscard"
            n119 = Variant To Data(error in=w172, type=dbl[] [] ("Position"), Variant=w175) -> (data=w174:dbl[], error out=w171:errorcluster)
            n120 = call <instrlib>:"MoveRel_all.vi"("# axis"=w178, "error in (no error)"=w171, "Position"=w174, "VISA resource name"=w177) -> ("error out"=w179:errorcluster)  [unwired: 7 in]
          }
          frame "Origin/Home" {
            n121 = call <instrlib>:"OriginSearch.vi"("HomeMode"=string[] ["4", "4", "4"], "#Axis"=w185, "error in"=w183, "VISA resource"=w184) -> ("error out"=w182:errorcluster)  [unwired: 7 in]
          }
          frame "WaitStop" {
            # "Wait stop  need refine to speed up \nserial communication"
            n122 = call <instrlib>:"WaitStop.vi"("error in (no error)"=w196, "VISA resource name"=w194) -> ("error out"=w195:errorcluster)  [unwired: 9 in]
            n123 = Variant To Data(type=refnum<queue> refnum ("Feedback"), Variant=w193) -> (data=w191:refnum<queue>)  [unwired: 1 in, 1 out]
            n124 = Enqueue Element(queue=w191, element="Done", error in (no error)=w195) -> (error out=w188:errorcluster)  [unwired: 1 in, 2 out]
            n125 = call <vilib>:"Clear Errors.vi"("error in (no error)"=w188) -> ("error out"=w189:errorcluster)  [unwired: 6 in]
          }
          frame "SetVelocity" {
            n126 = Variant To Data(error in=w207, type=cluster{"Axis":i32, "Velocity":dbl} {"Axis"=0, "Velocity"=0.0}, Variant=w208) -> (data=w202:cluster{"Axis":i32, "Velocity":dbl}, error out=w206:errorcluster)
            n127 = Unbundle By Name(w202) -> ("Axis"=w200:i32, "Velocity"=w201:dbl)
            n128 = call <instrlib>:"SetVelocity.vi"("error in"=w206, "Velocity"=w201, "Axial #"=w200, "VISA resource"=w209) -> ("error out"=w205:errorcluster)  [unwired: 7 in]
          }
          frame "SetAcceleration" {
            n129 = Variant To Data(error in=w219, type=cluster{"Axis":i32, "Acceleration":dbl} {"Axis"=0, "Acceleration"=0.0}, Variant=w220) -> (data=w214:cluster{"Axis":i32, "Acceleration":dbl}, error out=w218:errorcluster)
            n130 = Unbundle By Name(w214) -> ("Axis"=w213:i32, "Acceleration"=w212:dbl)
            n131 = call <instrlib>:"SetAcceleration.vi"("error in"=w218, "Acceleration"=w212, "Axial #"=w213, "VISA resource"=w221) -> ("error out"=w217:errorcluster)  [unwired: 7 in]
          }
          frame "GetVelocity" {
            # "to be written"
          }
          frame "GetAcceleration" {
            # "to be written"
          }
          frame "ClearErr" {
          }
          frame "LogMessage" {
          }
          frame "MotorEnable(1)" {
            n132 = Variant To Data(error in=w250, type=FALSE ("On/Off"), Variant=w248) -> (data=w244:bool, error out=w249:errorcluster)
            n133 = call <instrlib>:"MotorOnOff.vi"("#Axis"=w247, "error in"=w249, "Enabled"=w244, "VISA resource"=w246) -> ("error out"=w251:errorcluster)  [unwired: 7 in]
          }
          frame "JoyStick" {
            n134 = Variant To Data(type=cluster{"Axis":i32, "Speed":dbl} {"Axis"=0, "Speed"=0.0}, Variant=w262) -> (data=w260:cluster{"Axis":i32, "Speed":dbl})  [unwired: 1 in, 1 out]
            n135 = Unbundle By Name(w260) -> ("Axis"=w257:i32, "Speed"=w256:dbl)
            n136 = in-place {
              in-place-border: w259 -> [w271]
              in-place-border: [w270] -> w258
              in-place-border: w257 -> [w269]
              in-place-border: w256 -> [w268]
              in-place-border: w255 -> [w267]
              n137 = in-place-cluster #3(w254) -> ("JogSpeed"=w266:dbl[])
              n138 = call <instrlib>:"JoystickMove.vi"("JogSpeed"=w266, "error in"=w271, "Speed"=w268, "Axis"=w269, "ESP300"=w267) -> ("error out"=w270:errorcluster, "JogSpeed"=w265:dbl[])  [unwired: 5 in]
              n139 = in-place-cluster #3("JogSpeed"=w265) -> (w253:T5)
            }
          }
          frame "STOP" {
            # "Need test. Does set velocity interfere core"
            n140 = Unbundle By Name(w276) -> ("Velocity"=w275:dbl[])
            n141 = for {
              N: w272 -> [_]
              tunnel: w275 -> [w286] mode=indexing
              shift-right: [w285] -> _
              shift-left: w277 -> [w287]
              shift-right: [w284] -> w274
              shift-left: w273 -> [w283]
              i -> [w293]
              n142 = Increment(x=w293) -> (x+1=w291:i32)
              n143 = Bundle By Name(cluster=cluster{"Axis":i32, "Velocity":dbl} {"Axis"=0, "Velocity"=0.0}, "Velocity"=w286, "Axis"=w291) -> (w288:cluster{"Axis":i32, "Velocity":dbl})
              n144 = Bundle By Name(cluster=T3 {"State"=enum."SetVelocity", "Params."=variant} ("element"), "Params."=w288) -> (w290:T3)
              n145 = Enqueue Element(queue=w287, element=w290, error in (no error)=w283) -> (queue out=w285:refnum<queue>, error out=w284:errorcluster)  [unwired: 1 in, 1 out]
            }
            n146 = Initialize Array(0.0 ("element"), w272) -> (w278:dbl[])
            n147 = Bundle By Name(cluster=w276, "JogSpeed"=w278) -> (w280:T5)
          }
          frame Default {
            n148 = Unbundle By Name(w298) -> ("State"=w296:T12)
            n149 = Format Into String(format string="\nerror command %d", initial string="Error, no stop should be performed\nin blocking motion loop\nrefer to motion loop, Default frame" ("message"), w296) -> (resulting string=w297:string)  [unwired: 1 in, 1 out]
            n150 = One Button Dialog(message=w297) -> ()  [unwired: 1 in, 1 out]
          }
        }
        n151 = call <vilib>:"Clear Errors.vi"("error in (no error)"=w80) -> ("error out"=w67:errorcluster)  [unwired: 6 in]
        n152 = call <vilib>:"General Error Handler.vi"("type of dialog (OK msg:1)"=w73, "error in (no error)"=w67) -> ("error out"=w74:errorcluster)  [unwired: 9 in, 4 out]
      }
      n153 = Merge Errors(w55, w52) -> (w51:errorcluster)
    }
    frame True {
      n154 = while {
        tunnel: w496 -> [w804]
        shift-right: [w814] -> _
        shift-left: w497 -> [w813]
        tunnel: w495 -> [w811]
        shift-right: [w799] -> w489
        shift-left: w490 -> [w800]
        tunnel: 0 ("f") -> [w802]
        shift-right: [w798] -> _
        shift-left: T7 {"Position_Target"=[], "Velocity_axial"=[], "Acceleration"=[], "Moving"=FALSE, "Simulation"=FALSE, "tick_MoveTarget"=0, "NumOfAxis"=0, "Range"=[]} ("output cluster") -> [w797]
        stop <- w812 stop-if-true
        # "Unblocking loop"
        # "Non-blocking command Loop"
        n155 = Dequeue Element(queue=w804, timeout in ms (-1)=w802) -> (queue out=w805:refnum<queue>, element=w807:T3, timed out?=w809:bool, error out=w810:errorcluster)  [unwired: 1 in]
        n156 = Select(t=T8 {"State"=enum."UpdateXPos", "Params."=variant} ("element"), s=w809, f=w807) -> (s? t:f=w806:T3)
        n157 = Merge Errors(w810, w800) -> (w801:errorcluster)
        n158 = Unbundle By Name(w806) -> ("State"=w803:T12)
        n159 = case shown="\"GetVelocity\", \"GetAcceleration\"" w803 {
          tunnel: w806 -> [w826 w841 _ _ w904 w917 _ _ _ w995 w1012 w1018]
          tunnel: [w817 w838 w859 w883 w909 w913 w939 w970 w989 w998 w1002 w1023] -> w814
          tunnel: w813 -> [w828 w836 w859 w881 w900 w913 w937 w968 w989 w998 w1013 w1023]
          tunnel: [_ _ TRUE _ _ _ _ _ _ _ _ _] -> w812
          tunnel: w811 -> [w825 w842 w862 w888 w901 _ _ _ _ w997 _ w1022]
          tunnel: [w827 w839 w864 w886 w902 w915 w931 w969 errorcluster {"status"=FALSE, "code"=0, "source"=""} ("error out") w994 w1006 w1015] -> w799
          tunnel: w801 -> [w831 w840 w860 w887 w903 w916 w938 w969 _ w996 w1007 w1021]
          tunnel: w805 -> [_ w834 _ _ _ _ w930 _ _ _ _ w1019]
          tunnel: [w818 w833 w857 w884 w908 w911 w926 w966 w987 w990 w1005 w1014] -> w798
          tunnel: w797 -> [w824 w833 w857 w885 w910 w911 w926 w966 w987 w990 w1008 w1014]
          frame "Initialize" {
            # "cmd +(stage data)"
            # "stage data"
            n160 = Unbundle By Name(w826) -> ("Params."=w832:variant)
            n161 = Variant To Data(error in=w831, type=w828, Variant=w832) -> (data=w829:T4, error out=w830:errorcluster)
            n162 = Select(t=w828, s=w830, f=w829) -> (s? t:f=w820:T4)
            n163 = call <vilib>:"Clear Errors.vi"("error in (no error)"=w830) -> ("error out"=w827:errorcluster)  [unwired: 6 in]
            n164 = Unbundle By Name(w820) -> ("NumOfAxis"=w819:i32)
            n165 = Initialize Array(-1.2345 ("element"), w819) -> (w816:dbl[])
            n166 = global write "Position_ESP300.vi" "Position_ESP"(w816) -> ()
            n167 = Bundle By Name(cluster=w824, "Position_Target"=w816) -> (w818:T7)
            n168 = Bundle By Name(cluster=w820, "Position"=w816, "Initialized"=TRUE) -> (w817:T4)
            n169 = Bundle By Name(cluster=T8 {"State"=enum."Initialize", "Params."=variant}, "Params."=w820) -> (w823:T8)
            n170 = Enqueue Element(queue=w825, element=w823) -> ()  [unwired: 2 in, 3 out]
          }
          frame "Close" {
            n171 = Unbundle By Name(w836) -> ("Moving"=w835:bool)
            n172 = case shown="True" w835 {
              tunnel: w842 -> [w846 _]
              tunnel: w841 -> [w845 w847]
              tunnel: w840 -> [w844 w851]
              tunnel: [w843 w848] -> w839
              tunnel: w834 -> [_ w856]
              frame False {
                n173 = Enqueue Element(queue=w846, element=w845, error in (no error)=w844) -> (error out=w843:errorcluster)  [unwired: 1 in, 2 out]
              }
              frame True {
                n174 = Enqueue Element At Opposite End(queue=w856, element=w847, error in (no error)=w851) -> (queue out=w855:refnum<queue>, error out=w850:errorcluster)  [unwired: 1 in, 1 out]
                n175 = Enqueue Element At Opposite End(queue=w855, element=T8 {"State"=enum."UpdateAll", "Params."=variant}, error in (no error)=w850) -> (queue out=w854:refnum<queue>, error out=w849:errorcluster)  [unwired: 1 in, 1 out]
                n176 = Enqueue Element At Opposite End(queue=w854, element=T8 {"State"=enum."STOP", "Params."=variant}, error in (no error)=w849) -> (error out=w848:errorcluster)  [unwired: 1 in, 2 out]
              }
            }
            n177 = Bundle By Name(cluster=w836, "Initialized"=FALSE) -> (w838:T4)
          }
          frame "Quit" {
            n178 = Unbundle By Name(w859) -> ("Initialized"=w858:bool)
            n179 = case shown="False" w858 {
              tunnel: [w868 w872] -> w863
              tunnel: w862 -> [w868 w871]
              tunnel: [w867 w870] -> w861
              tunnel: w860 -> [w867 w869]
              frame False {
              }
              frame True {
                n180 = Enqueue Element(queue=w871, element=T8 {"State"=enum."Close", "Params."=variant}, error in (no error)=w869) -> (queue out=w872:refnum<queue>, error out=w870:errorcluster)  [unwired: 1 in, 1 out]
              }
            }
            n181 = Enqueue Element(queue=w863, element=T8 {"State"=enum."Quit", "Params."=variant}, error in (no error)=w861) -> (error out=w864:errorcluster)  [unwired: 1 in, 2 out]
          }
          frame "STOP" {
            w877 = T13 [enum."WaitStop", enum."UpdateAll", enum."Close", enum."Quit"] items=["Initialize", "SetDefaultConfig", "Close", "Quit", "Identify", "MoveAbs", "MoveAbs_all", "MoveRel", "MoveRel_all", "STOP", "Origin/Home", "WaitStop", "QueryStatus", "UpdateXPos", "UpdateAll", "SetVelocity", "SetAcceleration", "ClearErr", "LogMessage", "MotorEnable(1)", "EnableAxis", "JoyStick", "GetVelocity", "GetAcceleration", "SendCmd", "SetSoftLimits", "Beep", "_SettingReturn"]
            # "should not dump wait for stop!!"
            # "send stop to controller, update"
            n182 = Flush Queue(queue=w888, error in (no error)=w887) -> (queue out=w876:refnum<queue>, remaining elements=w875:T3[], error out=w886:errorcluster)
            n183 = for {
              tunnel: w875 -> [w895] mode=indexing
              tunnel: w877 -> [w892]
              shift-right: [w889] -> w874
              shift-left: w876 -> [w894]
              n184 = Unbundle By Name(w895) -> ("State"=w893:T12)
              n185 = Equal?(x=w893, y=w892) -> (x = y?=w890:bool[])
              n186 = Or Array Elements(Boolean array=w890) -> (logical OR=w891:bool)
              n187 = case shown="True" w891 {
                tunnel: w895 -> [_ w899]
                tunnel: w894 -> [w896 w898]
                tunnel: [w896 w897] -> w889
                frame False {
                }
                frame True {
                  n188 = Enqueue Element At Opposite End(queue=w898, element=w899) -> (queue out=w897:refnum<queue>)  [unwired: 2 in, 2 out]
                }
              }
            }
            n189 = Unbundle By Name(w881) -> ("Position"=w880:dbl[])
            n190 = Tick Count (ms)() -> (millisecond timer value=w879:u32)
            n191 = Bundle By Name(cluster=w885, "tick_MoveTarget"=w879, "Position_Target"=w880) -> (w884:T7)
            n192 = Bundle By Name(cluster=w881, "Position"=w880, "Moving"=FALSE) -> (w883:T4)
            n193 = Enqueue Element At Opposite End "Has to be PUSH"(queue=w874, element=T3 {"State"=enum."STOP", "Params."=variant}) -> ()  [unwired: 2 in, 3 out]
          }
          frame "Origin/Home" {
            n194 = Enqueue Element(queue=w901, element=w904, error in (no error)=w903) -> (error out=w902:errorcluster)  [unwired: 1 in, 2 out]
            n195 = Unbundle By Name(w900) -> ("NumOfAxis"=w907:i32)
            n196 = Initialize Array(0.0 ("element"), w907) -> (w905:dbl[])
            n197 = Bundle By Name(cluster=w910, "Position_Target"=w905) -> (w908:T7)
            n198 = Bundle By Name(cluster=w900, "Position"=w905) -> (w909:T4)
          }
          frame "QueryStatus" {
            # "return the value to queue"
            n199 = Unbundle By Name(w917) -> ("Params."=w919:variant)
            n200 = Variant To Data(error in=w916, type=refnum<queue> refnum ("queue out"), Variant=w919) -> (data=w914:refnum<queue>, error out=w918:errorcluster)
            n201 = Enqueue Element(queue=w914, element=w913, error in (no error)=w918) -> (error out=w915:errorcluster)  [unwired: 1 in, 2 out]
          }
          frame "UpdateXPos" {
            # "target position - (target tickcount - current tickcount)*velocity = current position"
            n202 = Unbundle By Name(w926) -> ("Position_Target"=w925:dbl[], "tick_MoveTarget"=w921:u32, "Velocity_axial"=w927:dbl[])
            n203 = feedback #4(0) -> (w934:i32)
            n204 = Increment(x=w934) -> (x+1=w935:i32)
            n205 = Quotient & Remainder(x=w935, y=16) -> (x-y*floor(x/y)=w932:i32)  [unwired: 1 out]
            n206 = feedback-in #4(w932) -> ()
            n207 = Wait (ms) "Typical latency of Micos Corvus PCI"(milliseconds to wait=u32 6) -> ()  [unwired: 1 out]
            n208 = Equal To 0?(x=w932) -> (x = 0?=w929:bool)
            n209 = Tick Count (ms)() -> (millisecond timer value=w922:u32)
            n210 = Less?(x=w922, y=w921) -> (x < y?=w923:bool)
            n211 = case shown="False" w923 {
              tunnel: [w944 w955] -> w939
              tunnel: w937 -> [w943 w954]
              tunnel: w921 -> [_ w953]
              tunnel: w927 -> [_ w951]
              tunnel: w925 -> [w941 w948]
              tunnel: w922 -> [w942 w947]
              tunnel: [w940 w945] -> w920
              frame False {
                w940 = FALSE ("Moving")
                # "Stopped"
                n212 = global write "Position_ESP300.vi" "Moving"(w940) -> ()
                n213 = global write "Position_ESP300.vi" "Position_ESP"(w941) -> ()
                n214 = Bundle By Name(cluster=w943, "tickcount_pos"=w942, "Position"=w941, "Moving"=w940) -> (w944:T4)
              }
              frame True {
                w945 = TRUE ("Moving")
                # "Moving"
                n215 = Subtract(x=w953, y=w947) -> (x-y=w952:u32)
                n216 = Compound Arithmetic op=MULTIPLY(w952, w951, 0.001) -> (w949:dbl[])
                n217 = Subtract(x=w948, y=w949) -> (x-y=w946:dbl[])
                n218 = global write "Position_ESP300.vi" "Moving"(w945) -> ()
                n219 = Bundle By Name(cluster=w954, "tickcount_pos"=w947, "Position"=w946, "Moving"=w945) -> (w955:T4)
                n220 = global write "Position_ESP300.vi" "Position_ESP"(w946) -> ()
              }
            }
            n221 = Compound Arithmetic op=OR(invert w920, w929) -> (w928:bool)
            n222 = case shown="True" w928 {
              tunnel: [w956 w960] -> w931
              tunnel: w930 -> [_ w959]
              tunnel: w938 -> [w956 w957]
              frame False {
              }
              frame True {
                n223 = Enqueue Element At Opposite End(queue=w959, element=T8 {"State"=enum."UpdateAll", "Params."=variant}, error in (no error)=w957) -> (error out=w960:errorcluster)  [unwired: 1 in, 2 out]
              }
            }
          }
          frame "UpdateAll" {
            # "target position - (target tickcount - current tickcount)*velocity = current position"
            n224 = Unbundle By Name(w966) -> ("Position_Target"=w965:dbl[], "tick_MoveTarget"=w961:u32, "Velocity_axial"=w967:dbl[])
            n225 = Wait (ms) "Typical latency of Micos Corvus PCI"(milliseconds to wait=u32 6) -> ()  [unwired: 1 out]
            n226 = Tick Count (ms)() -> (millisecond timer value=w962:u32)
            n227 = Greater Or Equal?(x=w962, y=w961) -> (x >= y?=w963:bool)
            n228 = case shown="False" w963 {
              tunnel: [w981 w986] -> w970
              tunnel: w968 -> [w980 w985]
              tunnel: w961 -> [w979 _]
              tunnel: w967 -> [w977 _]
              tunnel: w965 -> [w974 w983]
              tunnel: w962 -> [w973 w984]
              frame False {
                # "Generate current position"
                n229 = Subtract(x=w979, y=w973) -> (x-y=w978:u32)
                n230 = Compound Arithmetic op=MULTIPLY(w978, w977, 0.001) -> (w975:dbl[])
                n231 = Subtract(x=w974, y=w975) -> (x-y=w972:dbl[])
                n232 = Bundle By Name(cluster=w980, "tickcount_pos"=w973, "Position"=w972) -> (w981:T4)
                n233 = global write "Position_ESP300.vi" "Position_ESP"(w972) -> ()
                n234 = global write "Position_ESP300.vi" "Moving"(TRUE ("Moving")) -> ()
              }
              frame True {
                n235 = global write "Position_ESP300.vi" "Position_ESP"(w983) -> ()
                n236 = Bundle By Name(cluster=w985, "tickcount_pos"=w984, "Position"=w983) -> (w986:T4)
                n237 = global write "Position_ESP300.vi" "Moving"(FALSE ("Moving")) -> ()
              }
            }
          }
          frame "ClearErr" {
          }
          frame "GetVelocity", "GetAcceleration" {
            # "system does not response \nafter a command is received"
            # "timeout push command back then do update?\n\npreventing blocking"
            n238 = Enqueue Element(queue=w997, element=w995, error in (no error)=w996) -> (queue out=w992:refnum<queue>, error out=w991:errorcluster)  [unwired: 1 in, 1 out]
            n239 = Enqueue Element(queue=w992, element=T8 {"State"=enum."_SettingReturn", "Params."=variant}, error in (no error)=w991) -> (error out=w994:errorcluster)  [unwired: 1 in, 2 out]
          }
          frame "_SettingReturn" {
            n240 = Unbundle By Name(w1012) -> ("Params."=w1011:variant)
            n241 = Variant To Data(error in=w1007, type=T6 {"Acceleration"=[], "Velocity"=[], "tick_move_target"=0, "Position target"=[], "Velocity_axial"=[]}, Variant=w1011) -> (data=w1009:T6, error out=w1006:errorcluster)
            n242 = Unbundle By Name(w1009) -> ("Position target"=w1004:dbl[], "Velocity_axial"=w1003:dbl[], "tick_move_target"=w999:u32, "Velocity"=w1001:dbl[], "Acceleration"=w1000:dbl[])
            n243 = Bundle By Name(cluster=w1008, "Position_Target"=w1004, "Velocity_axial"=w1003, "tick_MoveTarget"=w999) -> (w1005:T7)
            n244 = Bundle By Name(cluster=w1013, "Velocity"=w1001, "Acceleration"=w1000) -> (w1002:T4)
          }
          frame Default {
            # "system does not response \nafter a command is received"
            # "timeout push command back then do update?\n\npreventing blocking"
            n245 = Enqueue Element(queue=w1022, element=w1018, timeout in ms (-1)=0, error in (no error)=w1021) -> (timed out?=w1016:bool, error out=w1017:errorcluster)  [unwired: 1 out]
            n246 = case shown="True" w1016 {
              tunnel: w1019 -> [_ w1031]
              tunnel: w1018 -> [_ w1030]
              tunnel: w1017 -> [w1024 w1029]
              tunnel: [w1024 w1026] -> w1015
              frame False {
              }
              frame True {
                n247 = Enqueue Element At Opposite End(queue=w1031, element=w1030, error in (no error)=w1029) -> (queue out=w1028:refnum<queue>, error out=w1025:errorcluster)  [unwired: 1 in, 1 out]
                n248 = Enqueue Element At Opposite End(queue=w1028, element=T8 {"State"=enum."UpdateXPos", "Params."=variant}, error in (no error)=w1025) -> (error out=w1026:errorcluster)  [unwired: 1 in, 2 out]
              }
            }
          }
        }
      }
      n249 = while {
        tunnel: w495 -> [w513]
        shift-right: [w510] -> w487
        shift-left: w494 -> [w511]
        shift-right: [w512] -> _
        shift-left: refnum<visa-resource-name> refnum ("CommPort") -> [w514]
        shift-right: [w520] -> _
        shift-left: _ -> [w519]
        shift-right: [w516] -> _
        shift-left: FALSE -> [w517]
        tunnel: w496 -> [w509]
        shift-right: [w508] -> _
        shift-left: T6 {"Acceleration"=[], "Velocity"=[], "tick_move_target"=0, "Position target"=[], "Velocity_axial"=[]} -> [w507]
        stop <- w522 stop-if-true
        w504 = T11 0 items=["no dialog", "OK message", "continue or stop message", "OK message + warnings", "continue/stop + warnings"] ("type of dialog (OK msg:1)")
        w505 = 1 items=["no exception", "cancel error on match", "set error on match"] ("[exception action] (none:0)")
        # "Blocking Comand Loop"
        n250 = Dequeue Element(queue=w513) -> (queue out=w500:refnum<queue>, element=w515:T3, error out=w521:errorcluster)  [unwired: 2 in, 1 out]
        n251 = Unbundle By Name(w515) -> ("Params."=w518:variant, "State"=w501:T12)
        n252 = Merge Errors(w521, w511) -> (w502:errorcluster)
        n253 = case "Exeacuting commands" shown="\"MoveRel_all\"" w501 {
          tunnel: w515 -> [w541 _ _ _ _ _ _ _ _ _ _ _ _ _ _ _ _ _ _ _ _ _ w792]
          tunnel: [_ _ _ TRUE _ _ _ _ _ _ _ _ _ _ _ _ _ _ _ _ _ _ _] -> w522
          tunnel: [w526 w545 w551 w556 w560 w572 w593 w619 w640 w659 w674 w677 w717 w733 errorcluster {"status"=FALSE, "code"=0, "source"=""} ("error out") w747 w753 w762 w768 w772 w777 w780 w795] -> w503
          tunnel: w502 -> [w539 w545 w551 w556 w560 w577 w603 w624 w650 w660 w674 w678 w718 w734 _ w747 w754 w759 w768 w772 w777 w779 w795]
          tunnel: [w536 w544 refnum<visa-resource-name> refnum ("CommPort") w555 w559 w579 w607 w626 w654 w666 w673 w688 w720 w736 w741 w746 w750 w757 w767 w771 w776 w787 w796] -> w512
          tunnel: w514 -> [_ w544 _ w555 w559 w579 w607 w626 w654 w666 w673 w688 w720 w736 w741 w746 w750 w757 w767 w771 w776 w787 w796]
          tunnel: w500 -> [w529 _ _ _ _ w571 w595 w618 w642 w662 _ w676 _ _ _ _ _ _ _ _ _ _ _]
          tunnel: [w523 w546 w549 w554 w562 w575 w608 w610 w655 w665 w668 w690 w712 w728 w740 w745 w751 w758 w766 w770 w775 w786 w794] -> w520
          tunnel: w519 -> [_ w546 w549 w554 w562 w575 w608 w610 w655 w665 w668 w690 w712 w728 w740 w745 w751 w758 w766 w770 w775 w786 w794]
          tunnel: w518 -> [_ _ _ _ _ w578 w605 w625 w652 _ _ w687 w719 w735 _ _ w752 w760 _ _ _ _ _]
          tunnel: w517 -> [_ w543 w548 w553 w561 w580 w606 w627 w653 w664 w672 w689 w716 w732 w739 w744 w755 w763 w765 w773 w778 w785 w793]
          tunnel: [w535 w543 w548 w553 w561 w580 w606 w627 w653 w664 w672 w689 w716 w732 w739 w744 w755 w763 w765 w773 w778 w785 w793] -> w516
          tunnel: w509 -> [_ _ _ _ _ _ _ _ _ _ _ _ _ _ _ _ _ _ _ _ _ w784 _]
          tunnel: [w533 w542 w547 w552 w558 w564 w601 w622 w648 w658 w670 w680 w714 w730 w738 w743 w748 w756 w764 w769 w774 w781 w788] -> w508
          tunnel: w507 -> [w534 w542 w547 w552 w558 w564 w602 w622 w649 w663 w671 w682 w711 w724 w738 w743 w748 w756 w764 w769 w774 w781 w788]
          frame "Initialize" {
            # "open port, set default config"
            n254 = Unbundle By Name(w541) -> ("Params."=w540:variant)
            n255 = Variant To Data(error in=w539, type=T9 {"Position"=[], "Velocity"=[], "Acceleration"=[], "Moving"=FALSE, "Simulation"=FALSE, "tickcount_mov"=0, "tickcount_pos"=0, "NumOfAxis"=0, "Initialized"=FALSE, "CommPort"="", "Range"=[], "Serial Configuration"={"Baud Rate"=0, "Parity"=0, "Data Bits"=0, "Stop Bits"=0, "Flow Control"=0}, "MotorDisabled"=refnum}, Variant=w540) -> (data=w537:T9, error out=w527:errorcluster)
            n256 = Unbundle By Name(w537) -> ("Simulation"=w535:bool, "NumOfAxis"=w523:i32, "CommPort"=w536:refnum<visa-resource-name>)
            n257 = Enqueue Element At Opposite End(queue=w529, element=T8 {"State"=enum."_SettingReturn", "Params."=variant}, error in (no error)=w527) -> (error out=w526:errorcluster)  [unwired: 1 in, 2 out]
            n258 = Tick Count (ms)() -> (millisecond timer value=w530:u32)
            n259 = Initialize Array(-1.2345 ("element"), w523) -> (w524:dbl[])
            n260 = Initialize Array(1.0 ("element"), w523) -> (w531:dbl[])
            n261 = Bundle By Name(cluster=w534, "Position target"=w524, "Acceleration"=w531, "Velocity"=w531, "tick_move_target"=w530) -> (w533:T6)
          }
          frame "SetDefaultConfig" {
          }
          frame "Close" {
          }
          frame "Quit" {
          }
          frame "Identify" {
          }
          frame "MoveAbs" {
            n262 = Variant To Data(error in=w577, type=cluster{"Axis":i32, "Position":dbl} {"Axis"=0, "Position"=0.0}, Variant=w578) -> (data=w569:cluster{"Axis":i32, "Position":dbl}, error out=w573:errorcluster)
            n263 = Unbundle By Name(w564) -> ("Position target"=w563:dbl[])
            n264 = Unbundle By Name(w569) -> ("Axis"=w568:i32, "Position"=w566:dbl)
            n265 = Decrement(x=w568) -> (x-1=w567:i32)
            n266 = in-place {
              in-place-border: w566 -> [w581]
              n267 = in-place-array #5(w563, w567) -> ()  [unwired: 1 out]
              n268 = in-place-array #5(w581) -> (w565:dbl[])  [unwired: 1 out]
            }
            n269 = Bundle By Name(cluster=T8 {"State"=enum."MoveAbs_all", "Params."=variant} ("element"), "Params."=w565) -> (w570:T8)
            n270 = Enqueue Element At Opposite End(queue=w571, element=w570, error in (no error)=w573) -> (error out=w572:errorcluster)  [unwired: 1 in, 2 out]
          }
          frame "MoveAbs_all" {
            n271 = global read "Position_ESP300.vi" "Position_ESP"() -> (w584:dbl[])
            n272 = Variant To Data(error in=w603, type=dbl[] [] ("Position"), Variant=w605) -> (data=w583:dbl[], error out=w594:errorcluster)
            n273 = Subtract(x=w583, y=w584) -> (x-y=w582:dbl[])
            n274 = Absolute Value(x=w582) -> (abs(x)=w586:dbl[])
            n275 = Unbundle By Name(w602) -> ("Velocity"=w589:dbl[])
            n276 = Array Max & Min(array=w586) -> (max value=w585:dbl)  [unwired: 3 out]
            n277 = Index Array(array=w589) -> (element=w588:dbl)  [unwired: 1 in]
            n278 = Reciprocal(x=w585) -> (1/x=w599:dbl)
            n279 = Reciprocal(x=w588) -> (1/x=w587:dbl)
            n280 = Enqueue Element At Opposite End(queue=w595, element=T8 {"State"=enum."_SettingReturn", "Params."=variant}, error in (no error)=w594) -> (error out=w593:errorcluster)  [unwired: 1 in, 2 out]
            n281 = Tick Count (ms)() -> (millisecond timer value=w596:u32)
            n282 = Compound Arithmetic op=MULTIPLY(w587, w585, 1000.0 ("value")) -> (w597:dbl)
            n283 = To Unsigned Long Integer(number=w597) -> (unsigned 32bit integer=w591:u32)
            n284 = Compound Arithmetic op=MULTIPLY(w589, w582, w599) -> (w600:dbl[])
            n285 = Add(x=w596, y=w591) -> (x+y=w598:u32)
            n286 = Bundle By Name(cluster=w602, "Position target"=w583, "Velocity_axial"=w600, "tick_move_target"=w598) -> (w601:T6)
          }
          frame "MoveRel" {
            n287 = Variant To Data(error in=w624, type=cluster{"Axis":i32, "Position":dbl} {"Axis"=0, "Position"=0.0}, Variant=w625) -> (data=w616:cluster{"Axis":i32, "Position":dbl}, error out=w620:errorcluster)
            n288 = Unbundle By Name(w616) -> ("Axis"=w615:i32, "Position"=w613:dbl)
            n289 = Initialize Array(0.0 ("element"), w610) -> (w609:dbl[])
            n290 = Decrement(x=w615) -> (x-1=w614:i32)
            n291 = in-place {
              in-place-border: w613 -> [w628]
              n292 = in-place-array #6(w609, w614) -> ()  [unwired: 1 out]
              n293 = in-place-array #6(w628) -> (w612:dbl[])  [unwired: 1 out]
            }
            n294 = Bundle By Name(cluster=T8 {"State"=enum."MoveRel_all", "Params."=variant} ("element"), "Params."=w612) -> (w617:T8)
            n295 = Enqueue Element At Opposite End(queue=w618, element=w617, error in (no error)=w620) -> (error out=w619:errorcluster)  [unwired: 1 in, 2 out]
          }
          frame "MoveRel_all" {
            n296 = global read "Position_ESP300.vi" "Position_ESP"() -> (w629:dbl[])
            n297 = Variant To Data(error in=w650, type=dbl[] [] ("Position"), Variant=w652) -> (data=w631:dbl[], error out=w641:errorcluster)
            n298 = Add(x=w629, y=w631) -> (x+y=w630:dbl[])
            n299 = Absolute Value(x=w631) -> (abs(x)=w633:dbl[])
            n300 = Array Max & Min(array=w633) -> (max value=w632:dbl)  [unwired: 3 out]
            n301 = Unbundle By Name(w649) -> ("Velocity"=w636:dbl[])
            n302 = Index Array(array=w636) -> (element=w635:dbl)  [unwired: 1 in]
            n303 = Reciprocal(x=w632) -> (1/x=w646:dbl)
            n304 = Reciprocal(x=w635) -> (1/x=w634:dbl)
            n305 = Tick Count (ms)() -> (millisecond timer value=w643:u32)
            n306 = Enqueue Element At Opposite End(queue=w642, element=T8 {"State"=enum."_SettingReturn", "Params."=variant}, error in (no error)=w641) -> (error out=w640:errorcluster)  [unwired: 1 in, 2 out]
            n307 = Compound Arithmetic op=MULTIPLY(w634, w632, 1000.0 ("value")) -> (w644:dbl)
            n308 = To Unsigned Long Integer(number=w644) -> (unsigned 32bit integer=w638:u32)
            n309 = Compound Arithmetic op=MULTIPLY(w636, w631, w646) -> (w647:dbl[])
            n310 = Add(x=w643, y=w638) -> (x+y=w645:u32)
            n311 = Bundle By Name(cluster=w649, "Position target"=w630, "Velocity_axial"=w647, "tick_move_target"=w645) -> (w648:T6)
          }
          frame "STOP" {
            # "Simulation only"
            # "Only for simulation, \nFor dumping the stop command left in queue."
            n312 = Enqueue Element At Opposite End(queue=w662, element=T8 {"State"=enum."_SettingReturn", "Params."=variant}, error in (no error)=w660) -> (error out=w659:errorcluster)  [unwired: 1 in, 2 out]
            n313 = global read "Position_ESP300.vi" "Position_ESP"() -> (w656:dbl[])
            n314 = Tick Count (ms)() -> (millisecond timer value=w657:u32)
            n315 = Bundle By Name(cluster=w663, "tick_move_target"=w657, "Position target"=w656) -> (w658:T6)
          }
          frame "Origin/Home" {
            n316 = Initialize Array(0.0 ("element"), w668) -> (w667:dbl[])
            n317 = Bundle By Name(cluster=w671, "Position target"=w667) -> (w670:T6)
          }
          frame "WaitStop" {
            n318 = Unbundle By Name(w682) -> ("tick_move_target"=w681:u32)
            n319 = Variant To Data(error in=w678, type=refnum<queue> refnum ("Feedback"), Variant=w687) -> (data=w685:refnum<queue>, error out=w675:errorcluster)
            n320 = while {
              tunnel: w676 -> [w691]
              tunnel: w681 -> [w703]
              tunnel: [w696] -> w679
              i -> [w695]
              stop <- w699 stop-if-true
              n321 = Preview Queue Element(queue=w691, timeout in ms (-1)=0) -> (element=w702:T3, timed out?=w692:bool)  [unwired: 1 in, 2 out]
              n322 = Unbundle By Name(w702) -> ("State"=w701:T12)
              n323 = Tick Count (ms)() -> (millisecond timer value=w704:u32)
              n324 = Equal?(x=T10."STOP" ("State"), y=w701) -> (x = y?=w697:bool)
              n325 = Greater Or Equal?(x=w704, y=w703) -> (x >= y?=w698:bool)
              n326 = Compound Arithmetic op=AND(w697, invert w692) -> (w693:bool)
              n327 = Select(t=w704, s=w693, f=w703) -> (s? t:f=w696:u32)
              n328 = Wait Until Next ms Multiple(millisecond multiple=u32 50) -> ()  [unwired: 1 out]
              n329 = Or(x=w698, y=w693) -> (x .or. y?=w699:bool)
              "WaitStopBlink" <- w695
            }
            n330 = Bundle By Name(cluster=w682, "tick_move_target"=w679) -> (w680:T6)
            n331 = Enqueue Element(queue=w685, element="Done", error in (no error)=w675) -> (error out=w683:errorcluster)  [unwired: 1 in, 2 out]
            n332 = call <vilib>:"Clear Errors.vi"("error in (no error)"=w683) -> ("error out"=w677:errorcluster)  [unwired: 6 in]
          }
          frame "SetVelocity" {
            n333 = Variant To Data(error in=w718, type=cluster{"Axis":i32, "Velocity":dbl} {"Axis"=0, "Velocity"=0.0}, Variant=w719) -> (data=w713:cluster{"Axis":i32, "Velocity":dbl}, error out=w717:errorcluster)
            n334 = Unbundle By Name(w711) -> ("Velocity"=w710:dbl[])
            n335 = Unbundle By Name(w713) -> ("Axis"=w708:i32, "Velocity"=w709:dbl)
            n336 = Decrement(x=w708) -> (x-1=w707:i32)
            n337 = in-place {
              in-place-border: w709 -> [w721]
              n338 = in-place-array #7(w710, w707) -> ()  [unwired: 1 out]
              n339 = in-place-array #7(w721) -> (w706:dbl[])  [unwired: 1 out]
            }
            n340 = Bundle By Name(cluster=w711, "Velocity"=w706) -> (w714:T6)
          }
          frame "SetAcceleration" {
            n341 = Variant To Data(error in=w734, type=cluster{"Axis":i32, "Acceleration":dbl} {"Axis"=0, "Acceleration"=0.0}, Variant=w735) -> (data=w729:cluster{"Axis":i32, "Acceleration":dbl}, error out=w733:errorcluster)
            n342 = Unbundle By Name(w729) -> ("Axis"=w723:i32, "Acceleration"=w722:dbl)
            n343 = Unbundle By Name(w724) -> ("Acceleration"=w727:dbl[])
            n344 = Decrement(x=w723) -> (x-1=w726:i32)
            n345 = in-place {
              in-place-border: w722 -> [w737]
              n346 = in-place-array #8(w727, w726) -> ()  [unwired: 1 out]
              n347 = in-place-array #8(w737) -> (w725:dbl[])  [unwired: 1 out]
            }
            n348 = Bundle By Name(cluster=w724, "Acceleration"=w725) -> (w730:T6)
          }
          frame "ClearErr" {
          }
          frame "LogMessage" {
          }
          frame "MotorEnable(1)" {
            n349 = Variant To Data(error in=w754, type=FALSE ("On/Off"), Variant=w752) -> (error out=w753:errorcluster)  [unwired: 1 out]
          }
          frame "EnableAxis" {
            n350 = Variant To Data(error in=w759, type=FALSE ("On/Off"), Variant=w760) -> (error out=w762:errorcluster)  [unwired: 1 out]
          }
          frame "JoyStick" {
          }
          frame "GetVelocity" {
            # "Send SettingReturn is taken cared in calling loop."
          }
          frame "GetAcceleration" {
            # "Send SettingReturn is taken cared in calling loop."
          }
          frame "_SettingReturn" {
            n351 = Bundle By Name(cluster=T8 {"State"=enum."_SettingReturn", "Params."=variant} ("element"), "Params."=w781) -> (w782:T8)
            n352 = Enqueue Element(queue=w784, element=w782, error in (no error)=w779) -> (error out=w780:errorcluster)  [unwired: 1 in, 2 out]
          }
          frame Default {
            n353 = Unbundle By Name(w792) -> ("State"=w790:T12)
            n354 = Format Into String(format string="\nUnsupported command:%d,\nDefault frame", w790) -> (resulting string=w791:string)  [unwired: 2 in, 1 out]
            n355 = One Button Dialog(message=w791) -> ()  [unwired: 1 in, 1 out]
          }
        }
        n356 = call <vilib>:"General Error Handler.vi"("type of dialog (OK msg:1)"=w504, "error in (no error)"=w503, "[exception action] (none:0)"=w505, "[exception code]"=-1073807339) -> ("error out"=w510:errorcluster)  [unwired: 7 in, 4 out]
      }
      n357 = Merge Errors(w489, w487) -> (w488:errorcluster)
    }
  }
  "error out" <- w2
  n358 = while {
    tunnel: w37 -> [w1034]
    tunnel: w10 -> [w1036]
    tunnel: w3 -> [w1032]
    tunnel: w25 -> [w1033]
    tunnel: [w1032] -> w1
    stop <- w1037 stop-if-true
    # "Control queue"
    n359 = event shown="[4] \"SetVelocity\": Value Change" {
      selector: _ -> [_ _ _ _ _ _ _ _ _ _ _ _ _]
      dyn-events: _ -> [_ _ _ _ _ _ _ _ _ _ _ _ _]
      timeout: 50 -> [_ _ _ _ _ _ _ _ _ _ _ _ _]
      tunnel: [w1038 _ _ _ _ _ _ _ _ _ _ TRUE _] -> w1037
      tunnel: w1036 -> [w1047 _ _ _ _ _ _ _ _ _ _ _ _]
      tunnel: w1034 -> [w1046 _ w1065 w1075 w1084 w1097 w1125 w1142 w1148 w1150 w1155 w1159 w1161]
      tunnel: w1032 -> [w1039 _ _ _ _ _ _ _ _ _ _ _ _]
      tunnel: w1033 -> [_ _ w1063 _ _ _ w1124 _ _ _ _ _ _]
      event Timeout {
        # "Send return queue ref"
        n360 = event-data() -> ()  [unwired: 1 in, 1 out]
        n361 = Not(x=w1047) -> (.not. x?=w1038:bool)
        n362 = Bundle By Name(cluster=T3 {"State"=enum."QueryStatus", "Params."=variant} ("element"), "Params."=w1039) -> (w1044:T3)
        n363 = Enqueue Element(queue=w1046, element=w1044) -> (error out=w1042:errorcluster)  [unwired: 2 in, 2 out]
        n364 = Dequeue Element(queue=w1039, timeout in ms (-1)=1000, error in (no error)=w1042) -> (element=w1040:T4, timed out?=w1041:bool)  [unwired: 2 out]
        n365 = case shown="True" w1041 {
          tunnel: w1040 -> [w1052 _]
          frame False {
            n366 = Unbundle By Name(w1052) -> ("Position"=→"Position":dbl[], "Velocity"=→"Velocity":dbl[], "Acceleration"=→"Acceleration":dbl[], "Moving"=→"Moving":bool)
          }
          frame True {
          }
        }
      }
      event "Position": Mouse Down {
        n367 = event-data() -> ("CtlRef"=w1054:refnum<vi>, "Mods.Double Click"=w1055:bool)  [unwired: 1 in]
        n368 = control-ref of="SetPosition"() -> (w1053:refnum<vi>)
        n369 = case shown="True" w1055 {
          tunnel: w1054 -> [_ w1059]
          tunnel: w1053 -> [_ w1058]
          frame False {
          }
          frame True {
            n370 = property class="Arr (strict)"(reference=w1059) -> (error out=w1057:errorcluster, "Value"=w1056:dbl[])  [unwired: 1 in, 1 out]
            n371 = property class="Arr (strict)"(reference=w1058, error in=w1057, "Value"=w1056) -> ()  [unwired: 2 out]
          }
        }
      }
      event "Go": Value Change {
        n372 = event-data() -> ()  [unwired: 1 in, 1 out]
        n373 = Unbundle By Name(w1063) -> ("SetPosition"=w1062:refnum<vi>)
        n374 = property class="Arr (strict)"(reference=w1062) -> ("Value"=w1060:dbl[])  [unwired: 1 in, 2 out]
        n375 = Bundle By Name(cluster=T3 {"State"=enum."MoveAbs_all", "Params."=variant} ("element"), "Params."=w1060) -> (w1061:T3)
        n376 = Enqueue Element(queue=w1065, element=w1061) -> ()  [unwired: 2 in, 3 out]
      }
      event "SetPosition": Value Change {
        n377 = event-data() -> ("OldVal"=w1072:dbl[], "NewVal"=w1071:dbl[])  [unwired: 1 in]
        n378 = for {
          tunnel: w1072 -> [w1079] mode=indexing
          tunnel: w1071 -> [w1076] mode=indexing
          tunnel: [w1078] -> w1070
          tunnel: [w1076] -> w1067
          i -> [w1078]
          stop <- w1077 continue-if-true
          n379 = Equal?(x=w1079, y=w1076) -> (x = y?=w1077:bool)
        }
        n380 = Increment(x=w1070) -> (x+1=w1068:i32)
        n381 = Bundle By Name(cluster=cluster{"Axis":i32, "Position":dbl} {"Axis"=0, "Position"=0.0}, "Position"=w1067, "Axis"=w1068) -> (w1066:cluster{"Axis":i32, "Position":dbl})
        n382 = Bundle By Name(cluster=T3 {"State"=enum."MoveAbs", "Params."=variant} ("element"), "Params."=w1066) -> (w1073:T3)
        n383 = Enqueue Element(queue=w1075, element=w1073) -> ()  [unwired: 2 in, 3 out]
      }
      event "SetVelocity": Value Change {
        n384 = event-data() -> ("NewVal"=w1083:dbl[])  [unwired: 1 in]
        n385 = property on="NumOfAxis" class="DigNum (strict)"() -> ("Value"=w1082:i32)  [unwired: 2 in, 2 out]
        n386 = for {
          N: w1082 -> [_]
          tunnel: w1083 -> [w1086] mode=indexing
          shift-right: [w1085] -> w1081
          shift-left: w1084 -> [w1087]
          i -> [w1093]
          n387 = Increment(x=w1093) -> (x+1=w1091:i32)
          n388 = Bundle By Name(cluster=cluster{"Axis":i32, "Velocity":dbl} {"Axis"=0, "Velocity"=0.0}, "Velocity"=w1086, "Axis"=w1091) -> (w1088:cluster{"Axis":i32, "Velocity":dbl})
          n389 = Bundle By Name(cluster=T3 {"State"=enum."SetVelocity", "Params."=variant} ("element"), "Params."=w1088) -> (w1090:T3)
          n390 = Enqueue Element(queue=w1087, element=w1090) -> (queue out=w1085:refnum<queue>)  [unwired: 2 in, 2 out]
        }
        n391 = Enqueue Element(queue=w1081, element=T3 {"State"=enum."GetVelocity", "Params."=variant}) -> ()  [unwired: 2 in, 3 out]
      }
      event "SetAcceleration": Value Change {
        n392 = event-data() -> ("NewVal"=w1098:dbl[])  [unwired: 1 in]
        n393 = property on="NumOfAxis" class="DigNum (strict)"() -> ("Value"=w1096:i32)  [unwired: 2 in, 2 out]
        n394 = for {
          N: w1096 -> [_]
          tunnel: w1098 -> [w1100] mode=indexing
          shift-right: [w1099] -> w1095
          shift-left: w1097 -> [w1101]
          i -> [w1107]
          n395 = Increment(x=w1107) -> (x+1=w1105:i32)
          n396 = Bundle By Name(cluster=cluster{"Axis":i32, "Acceleration":dbl} {"Axis"=0, "Acceleration"=0.0}, "Acceleration"=w1100, "Axis"=w1105) -> (w1102:cluster{"Axis":i32, "Acceleration":dbl})
          n397 = Bundle By Name(cluster=T3 {"State"=enum."SetAcceleration", "Params."=variant} ("element"), "Params."=w1102) -> (w1104:T3)
          n398 = Enqueue Element(queue=w1101, element=w1104) -> (queue out=w1099:refnum<queue>)  [unwired: 2 in, 2 out]
        }
        n399 = Enqueue Element(queue=w1095, element=T3 {"State"=enum."GetAcceleration", "Params."=variant}) -> ()  [unwired: 2 in, 3 out]
      }
      event "X+", "Y+", "Y-", "X-", "Z+", "Z-": Value Change {
        n400 = event-data() -> ()  [unwired: 1 in, 1 out]
        n401 = Unbundle By Name(w1124) -> ("StepWidth"=w1123:refnum<vi>)
        n402 = property class="Ring (strict)"(reference=w1123) -> ("Value"=w1114:T14)  [unwired: 1 in, 2 out]
        n403 = Build Array("X+", "X-", "Y+", "Y-", "Z+", "Z-") -> (w1122:bool[])
        n404 = Search 1D Array(1D array=w1122, element=TRUE) -> (index of element=w1119:i32)  [unwired: 1 in]
        n405 = Index Array(array=dbl[] [1.0, -1.0, 1.0, -1.0, 1.0, -1.0], index=w1119) -> (element=w1118:dbl)
        n406 = Index Array(array=i32[] [1, 1, 2, 2, 3, 3], index=w1119) -> (element=w1112:i32)
        n407 = Multiply(x=w1114, y=w1118) -> (x*y=w1113:T14)
        n408 = Bundle By Name(cluster=cluster{"Axis":i32, "Position":dbl} {"Axis"=0, "Position"=0.0}, "Position"=w1113, "Axis"=w1112) -> (w1126:cluster{"Axis":i32, "Position":dbl})
        n409 = Bundle By Name(cluster=T3 {"State"=enum."MoveRel", "Params."=variant} ("element"), "Params."=w1126) -> (w1128:T3)
        n410 = Enqueue Element(queue=w1125, element=w1128) -> ()  [unwired: 2 in, 3 out]
      }
      event "-Z", "+Z", "--Z", "++Z", "-Z_fine", "+Z_fine": Value Change {
        n411 = event-data() -> ()  [unwired: 1 in, 1 out]
        n412 = Build Array("--Z", "-Z", "-Z_fine", "+Z_fine", "+Z", "++Z") -> (w1138:bool[])
        n413 = Search 1D Array(1D array=w1138, element=TRUE) -> (index of element=w1135:i32)  [unwired: 1 in]
        n414 = Index Array(array=dbl[] [-0.1, -0.01, -0.001, 0.001, 0.01, 0.1], index=w1135) -> (element=w1134:dbl)
        n415 = Bundle By Name(cluster=cluster{"Axis":i32, "Position":dbl} {"Axis"=0, "Position"=0.0}, "Position"=w1134, "Axis"=3) -> (w1143:cluster{"Axis":i32, "Position":dbl})
        n416 = Bundle By Name(cluster=T3 {"State"=enum."MoveRel", "Params."=variant} ("element"), "Params."=w1143) -> (w1145:T3)
        n417 = Enqueue Element(queue=w1142, element=w1145) -> ()  [unwired: 2 in, 3 out]
      }
      event "STOP": Value Change {
        n418 = event-data() -> ()  [unwired: 1 in, 1 out]
        n419 = Enqueue Element(queue=w1148, element=T3 {"State"=enum."STOP", "Params."=variant}) -> ()  [unwired: 2 in, 3 out]
      }
      event "Home": Value Change {
        n420 = event-data() -> ()  [unwired: 1 in, 1 out]
        n421 = Enqueue Element(queue=w1150, element=T3 {"State"=enum."Origin/Home", "Params."=variant}) -> ()  [unwired: 2 in, 3 out]
      }
      event "MotorDisabled": Value Change {
        n422 = event-data() -> ()  [unwired: 1 in, 1 out]
        n423 = Not(x="MotorDisabled") -> (.not. x?=w1151:bool)
        n424 = Bundle By Name(cluster=T3 {"State"=enum."MotorEnable(1)", "Params."=variant} ("element"), "Params."=w1151) -> (w1153:T3)
        n425 = Enqueue Element(queue=w1155, element=w1153) -> ()  [unwired: 2 in, 3 out]
      }
      event "Quit": Value Change {
        n426 = event-data() -> ()  [unwired: 1 in, 1 out]
        n427 = property on="Quit" class="Bool (strict)"("Value"=FALSE ("Quit")) -> ()  [unwired: 2 in, 2 out]
        n428 = Enqueue Element(queue=w1159, element=T3 {"State"=enum."Quit", "Params."=variant}) -> ()  [unwired: 2 in, 3 out]
      }
      event "ClearErr": Value Change {
        n429 = event-data() -> ()  [unwired: 1 in, 1 out]
        n430 = Enqueue Element(queue=w1161, element=T3 {"State"=enum."ClearErr", "Params."=variant}) -> ()  [unwired: 2 in, 3 out]
      }
    }
  }
  n431 = Release Queue(queue=w4, error in (no error)=w2) -> ()  [unwired: 1 in, 3 out]
  n432 = Release Queue(queue=w1, error in (no error)=w2) -> ()  [unwired: 1 in, 3 out]
